vi "Main.vi"() -> ()   [LabVIEW 2019]
panel:
  out "status reference out":bool=TRUE
  in  "Find":bool
  in  "stop 2":bool
  in  "axis in":u8
  in  "stop":bool
  in  "Tab Control":enum32{"Navigation", "Interface", "About"}(tab)
  in  "find ref":bool
  in  "Reference Auto Update 3":bool=TRUE caption="Auto Update"
  out "move out":bool=TRUE caption="Move"
  in  "Positioner 2":u16(ring)=15 caption="Positioner" items=["ECGp5050", "ECGt5050", "ECR3030", "ECR4040", "ECR5050", "ECSx3030", "ECSx3040", "ECSx3050", "ECSx3060", "ECSx3070", "ECSx3080", "ECSx5050", "ECSxy5050", "ECSz3030", "ECSz5050", "EOP1", "EOP2", "EOP3"]
  out "in target range3":bool
  in  "auto Reset 1":bool=TRUE caption="Auto Reset"
  in  "Target Range 3":u32 caption="Target Range"
  in  "Reset Error 2":bool
  in  "Reset Error 3":bool
  out "Error 3":bool caption="Error"
  out "Error Message 3":string
  out "actor type 2":u16(ring) caption="Status" items=["linear positioner"=0, "rotator"=1, "goniometer"=2, "< error >"=9]
  out "actor type":u16(ring) caption="Status" items=["linear positioner"=0, "rotator"=1, "goniometer"=2, "< error >"=9]
  out "EotLeftDetected3":bool caption="Status Eot BWD"
  out "EotrightDetected3":bool caption="Status Eot FWD"
  in  "EoT 3":bool=TRUE caption="Stop on EoT"
  out "EotLeftDetected2":bool caption="Status Eot BWD"
  out "EotrightDetected2":bool caption="Status Eot FWD"
  in  "EoT 2":bool=TRUE caption="Stop on EoT"
  in  "Move 3":bool
  out "MoveSignal 3":bool caption="Positioner Connected/Moving"
  out "MoveSignal":bool caption="Positioner Connected/Moving"
  out "ReferenceSignal":bool=TRUE
  in  "Axis 3":bool caption="Closed Loop Funktions"
  in  "Axis 2":bool caption="Closed Loop Funktions"
  in  "Target Position 3":i32 caption="Target Position [µm]"
  in  "Target Position 1":i32 caption="Target position [µm]"
  in  "Number of steps 3":i32=1 caption="Number of Steps"
  in  "Number of steps 2":i32=1 caption="Number of Steps"
  in  "Output 2":bool caption="Axis 2"
  in  "Move 2":bool
  in  "Move":bool
  out "ReferenceSignal 3":bool
  out "Reference 3":dbl caption="Reference position [nm]" format="%#_6f"
  in  "Output":bool=TRUE caption="Axis 1"
  out "Output Satus 3":bool caption="Output Status"
  in  "Reference Auto Update 2":bool=TRUE caption="Auto Update"
  out "Error Message":string
  out "Error":bool
  in  "Output 3":bool caption="Axis 3"
  in  "auto Reset 3":bool=TRUE caption="Auto Reset"
  out "Output Status 1":bool=TRUE caption="Output Status"
  out "Position 3":dbl caption="Position [nm]" format="%#_6f"
  out "Output Status 2":bool caption="Output Status"
  in  "amplitude [V] 3":dbl=45.001 caption="Amplitude [V]" format="%#.3f"
  in  "frequency [Hz] 3":dbl=997.363 caption="Frequency [Hz]" format="%#.3f"
  out "Error 2":bool caption="Error"
  out "actor type 3":u16(ring) caption="Status" items=["linear positioner"=0, "rotator"=1, "goniometer"=2, "< error >"=9]
  out "Error Message 2":string
  out "Connected 3":bool caption="Connected"
  in  "Single Step Left 3":bool caption="Open Loop Funktions"
  in  "Positioner 3":u16(ring)=15 caption="Positioner" items=["ECGp5050", "ECGt5050", "ECR3030", "ECR4040", "ECR5050", "ECSx3030", "ECSx3040", "ECSx3050", "ECSx3060", "ECSx3070", "ECSx3080", "ECSx5050", "ECSxy5050", "ECSz3030", "ECSz5050", "EOP1", "EOP2", "EOP3"]
  in  "Endless Left 3":bool caption="Continuous Backward"
  in  "Continuous Forward":bool
  in  "Single Step Right 3":bool caption="Step(s)"
  in  "Fixed DC 3":i32 caption="DC Level [mV]"
  out "move out 3":bool=TRUE caption="Move"
  out "Position 2":dbl caption="Position [nm]" format="%#_6f"
  in  "amplitude [V] 2":dbl=45.001 caption="Amplitude [V]" format="%#.3f"
  in  "Amplitude [V]":dbl=45.001 format="%#.3f"
  in  "frequency [Hz] 2":dbl=997.363 caption="Frequency [Hz]" format="%#.3f"
  in  "Frequency [Hz]":dbl=1998.531 format="%#.3f"
  out "Connected 2":bool caption="Connected"
  in  "Single Step Left":bool caption="Open Loop Funktions"
  in  "Single Step Left 2":bool caption="Open Loop Funktions"
  in  "Single Step Right 2":bool caption="Step(s)"
  in  "Number of steps 1":i32=1 caption="Number of Steps"
  out "ReferenceSignal 2":bool
  in  "Single Step Right":bool caption="Step(s)"
  in  "Endless Left":bool caption="Continuous Backward"
  in  "Continuous Forward":bool
  in  "Endless Left 2":bool caption="Continuous Backward"
  out "EotLeftDetected1":bool caption="Status Eot BWD"
  out "EotrightDetected1":bool caption="Status Eot FWD"
  in  "EoT 1":bool caption="Stop on EoT"
  in  "Target position 2":i32 caption="Target Position [µm]"
  out "in target range2":bool
  in  "Continuous Forward":bool
  out "Reference 2":dbl caption="Reference position [nm]" format="%#_6f"
  in  "Fixed DC 2":i32 caption="DC Level [mV]"
  out "MoveSignal 2":bool caption="Positioner Connected/Moving"
  out "in target range1":bool
  in  "Target Range 2":u32 caption="Target Range [nm]"
  in  "Target Range 1":u32 caption="Target Range"
  out "Reference":dbl=-7597148.0 caption="Reference position [nm]" format="%#_6f"
  in  "auto Reset 2":bool=TRUE caption="Auto Reset"
  out "Position":dbl=14701.126 caption="Position [nm]" format="%#_6f"
  in  "Axis 1":bool caption="Closed Loop Funktions"
  in  "Fixed DC 1":i32 caption="DC Level [mV]"
  out "move out 2":bool=TRUE caption="Move"
  in  "Reset Error":bool
  out "Connected":bool=TRUE
  in  "Positioner":u16(ring)=15 items=["ECGp5050", "ECGt5050", "ECR3030", "ECR4040", "ECR5050", "ECSx3030", "ECSx3040", "ECSx3050", "ECSx3060", "ECSx3070", "ECSx3080", "ECSx5050", "ECSxy5050", "ECSz3030", "ECSz5050", "EOP1", "EOP2", "EOP3"]
  in  "Reference Auto Update 1":bool=TRUE caption="Auto Update"
  out "Voltage (mv)":i64
  out "Error 4":bool caption="Error"
  out "Error Message 4":string
  in  "Mode Input 1":u16(ring) caption="Mode" items=["Trigger (LVDS)"=11, "Trigger (LVTTL)"=10, "Stepper (LVDS)"=9, "Stepper (LVTTL)"=8, "AquadB (LVDS)"=1, "AquadB (LVTTL)"=0, "OFF"=15]
  in  "Loop Mode 1":u16(ring) caption="Loop mode" items=["closed-loop"=1, "open-loop"=0]
  in  "Steps per pulse 1":i32 caption="Steps per pulse [Steps]"
  in  "Change per pulse 1":i32 caption="Change per pulse [u°/nm]"
  out "RT in move Signal 1":bool=TRUE caption="move"
  in  "RT in move 1":bool=TRUE caption="Move"
  in  "AquadB in res 1":i32 caption="AquadB Resolution [nm]"
  in  "AquadB out 1":bool caption="AquadB enable"
  in  "AqaudB clock 1":i32 caption="AquadB Clock [ns]"
  in  "AquadB Resolution 1":i32 caption="AquadB Resolution [nm]"
  in  "Reset Error 4":bool
  out "Error 5":bool caption="Error"
  out "Error Message 5":string
  in  "Mode Input 2":u16(ring) caption="Mode" items=["Trigger (LVDS)"=11, "Trigger (LVTTL)"=10, "Stepper (LVDS)"=9, "Stepper (LVTTL)"=8, "AquadB (LVDS)"=1, "AquadB (LVTTL)"=0, "OFF"=15]
  in  "Loop Mode 2":u16(ring) caption="Loop mode" items=["closed-loop"=1, "open-loop"=0]
  in  "Steps per pulse 2":i32 caption="Steps per pulse [Steps]"
  in  "Change per pulse 2":i32 caption="Change per pulse  [u°/nm]"
  out "RT in move Signal 2":bool=TRUE caption="move"
  in  "RT in move 2":bool=TRUE caption="Move"
  in  "AquadB in res 2":i32 caption="AquadB Resolution [nm]"
  in  "AquadB out 2":bool caption="AquadB enable"
  in  "AqaudB clock 2":i32 caption="AquadB Clock [ns]"
  in  "AquadB Resolution 2":i32 caption="AquadB Resolution [nm]"
  in  "Reset Error 5":bool
  out "Error 6":bool caption="Error"
  out "Error Message 6":string
  in  "Mode Input 3":u16(ring) caption="Mode" items=["Trigger (LVDS)"=11, "Trigger (LVTTL)"=10, "Stepper (LVDS)"=9, "Stepper (LVTTL)"=8, "AquadB (LVDS)"=1, "AquadB (LVTTL)"=0, "OFF"=15]
  in  "Loop Mode 3":u16(ring) caption="Loop mode" items=["closed-loop"=1, "open-loop"=0]
  in  "Steps per pulse 3":i32 caption="Steps per pulse [Steps]"
  in  "Change per pulse 3":i32 caption="Change per pulse  [u°/nm]"
  out "RT in move Signal 3":bool=TRUE caption="move"
  in  "RT in move 3":bool=TRUE caption="Move"
  in  "AquadB in res 3":i32 caption="AquadB Resolution [nm]"
  in  "Output Mode":u16(ring) caption="Mode" items=["AquadB (LVTTL)", "AquadB (LVDS)"]
  in  "AquadB out 3":bool caption="AquadB enable"
  in  "AqaudB clock 3":i32 caption="AquadB Clock [ns]"
  in  "AquadB Resolution 3":i32 caption="AquadB Resolution [nm]"
  in  "Reset Error 6":bool
  in  "Reboot":bool
  in  "Factory Reset":bool
  in  "Reset Error 8":bool
  out "Error Message 7":string
  in  "Lock password":string
  in  "name":string="Test" caption="Device Name"
  in  "Access Password":string
  out "Error 7":bool caption="Error"
  out "locked":bool
  out "authorized":bool
  in  "Unlock":bool=TRUE
  out "Name":string caption="Device Name"
  out "Device type":string="AMC100/NUM"
  out "Sn":string caption="Serial Number"
  out "ip":string="192.168.1.1" caption="IP Adress"
  out "Firmware Version":string
  out "FPGA Version":string
  out "Mac Adress":string
  # "Real Time Input"
  # "Real Time Output"
  # "Global Parameters"
  # "Axis 1"
  # "Axis 1"
  # "Axis 2"
  # "Axis 2"
  # "Axis 3"
  # "Axis 3"
  # "Device Info"
  # "Device Access"
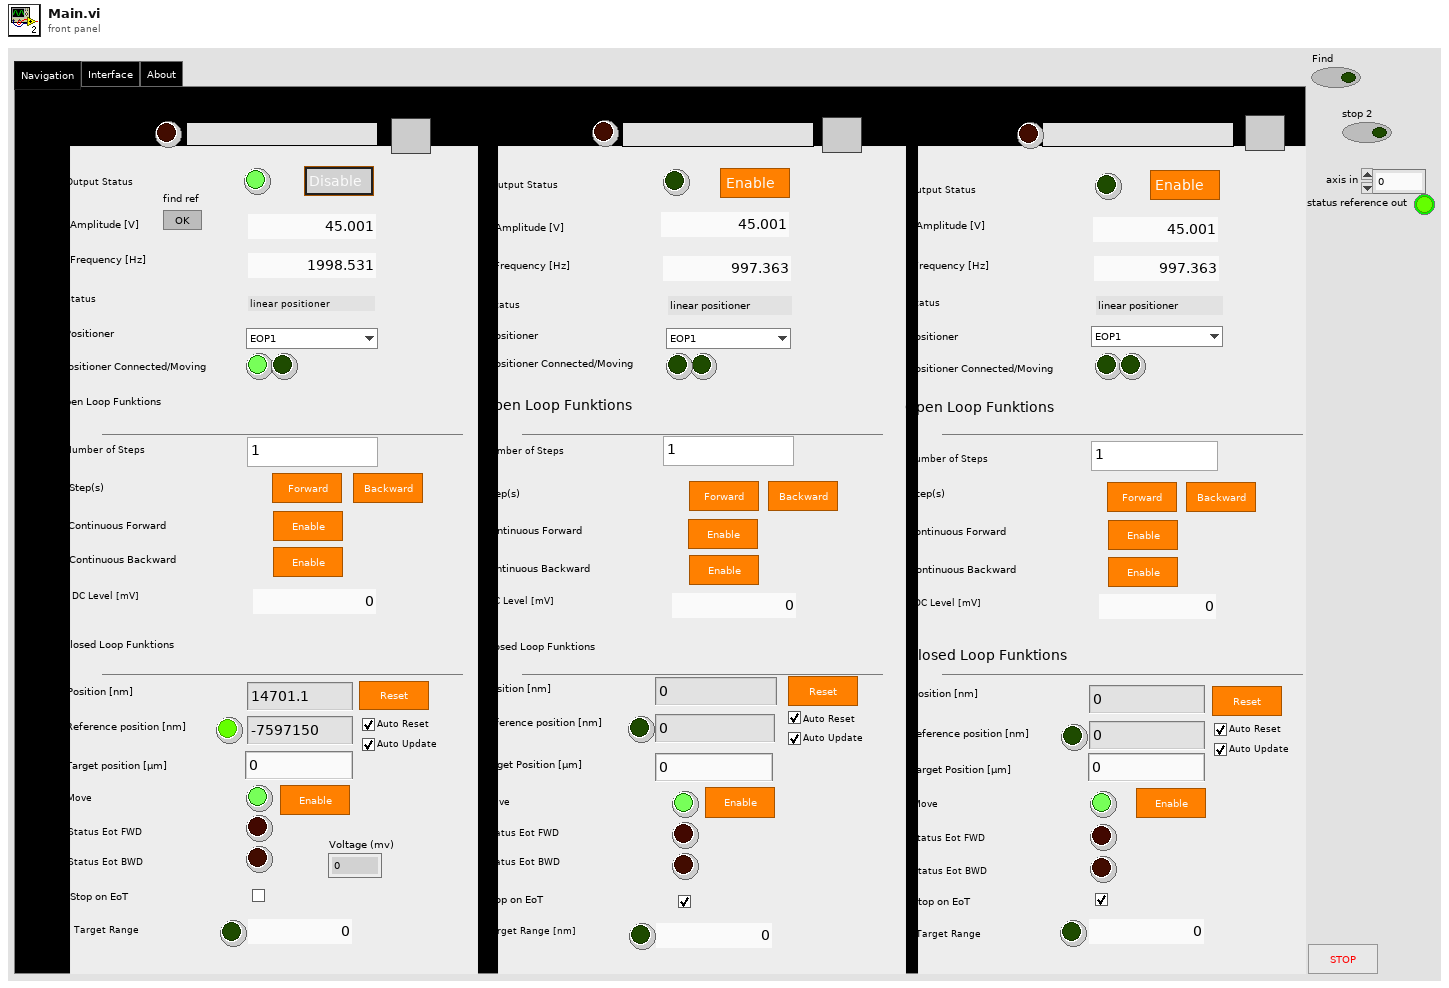
[diagram p1: front panel]
types:
  T1 = enum8{"Enabled", "Disabled", "Disabled and Grayed Out"}
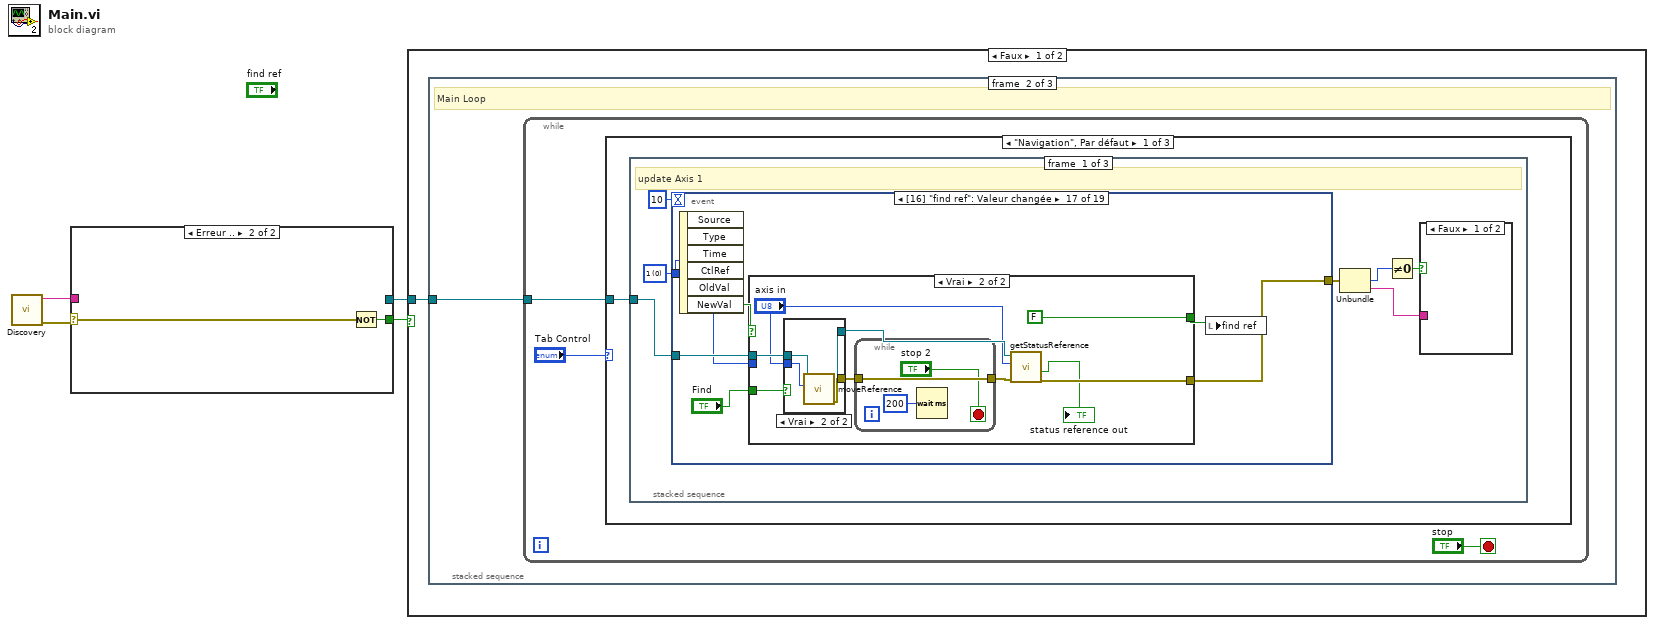
[diagram p0: block diagram]
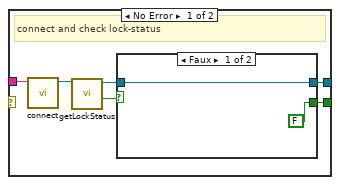
[diagram p2: hidden frame]
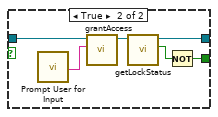
[diagram p3: hidden frame]
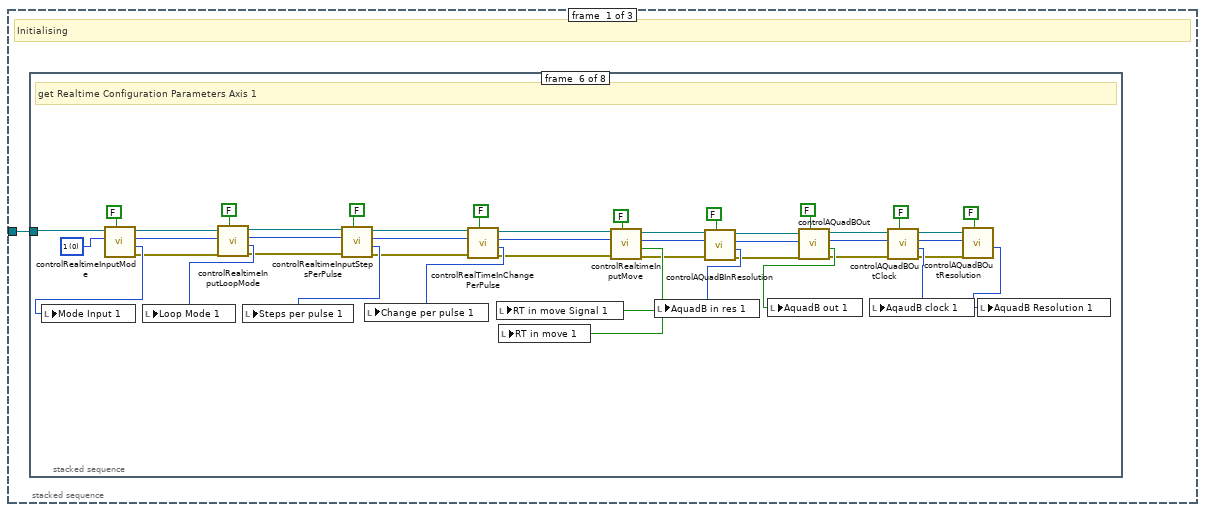
[diagram p4: hidden frame]
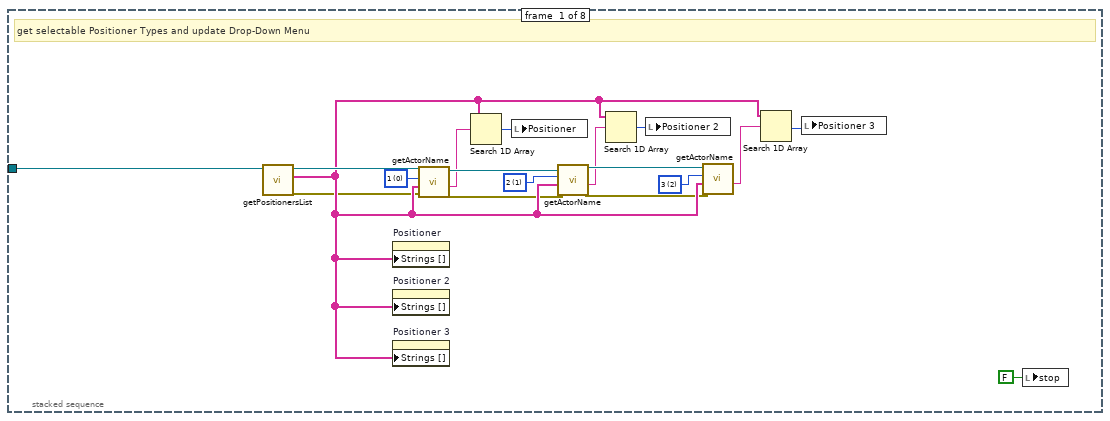
[diagram p5: hidden frame]
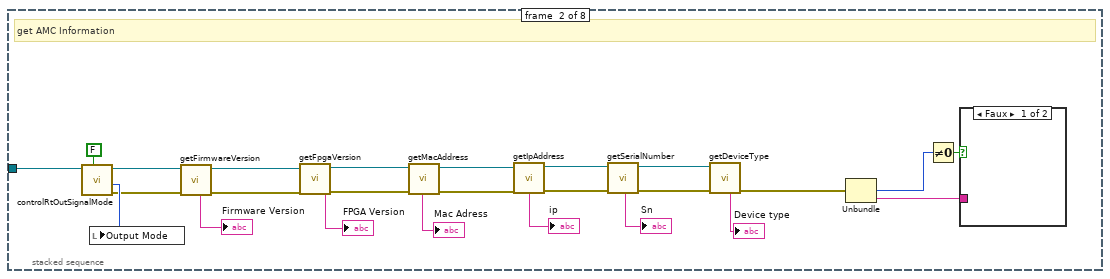
[diagram p6: hidden frame]
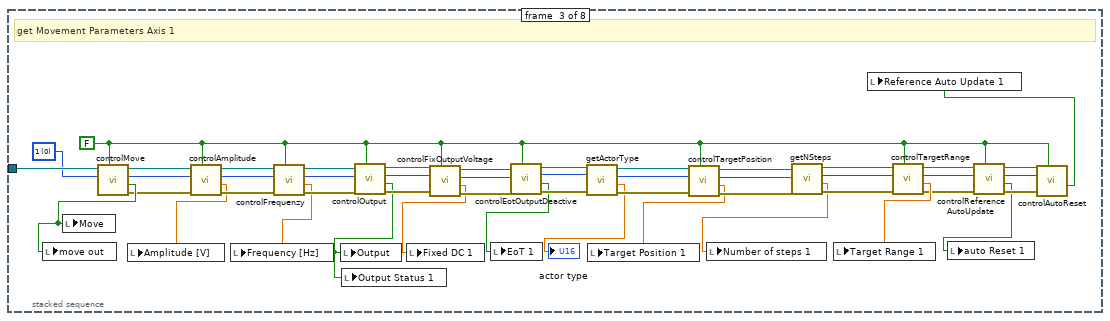
[diagram p8: hidden frame]
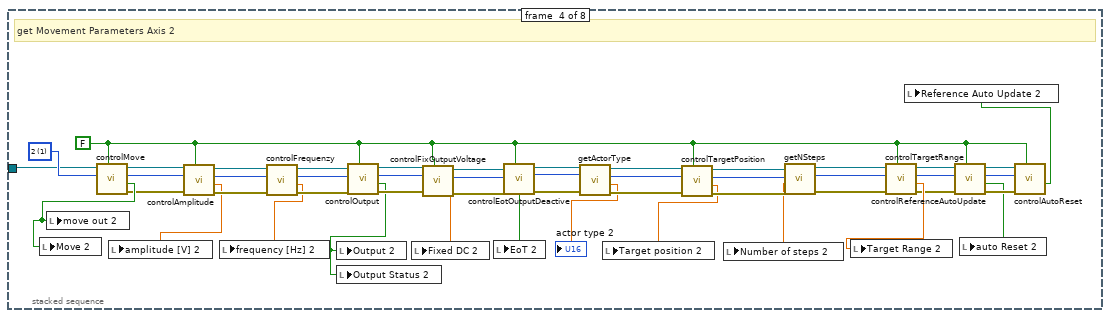
[diagram p9: hidden frame]
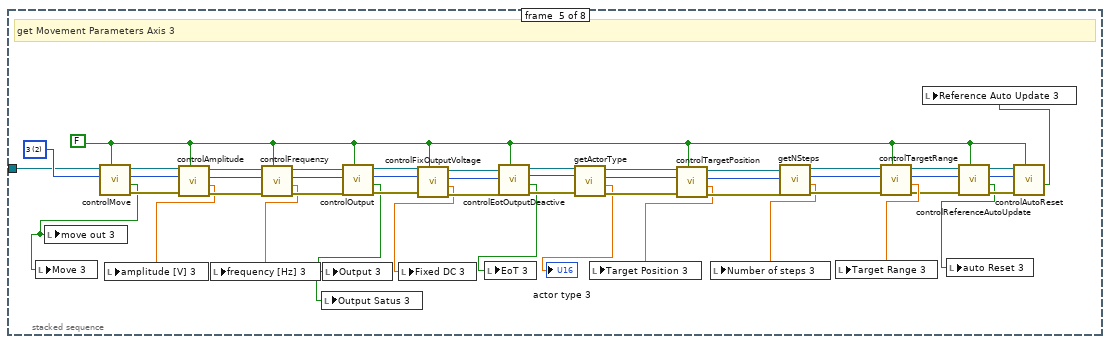
[diagram p10: hidden frame]
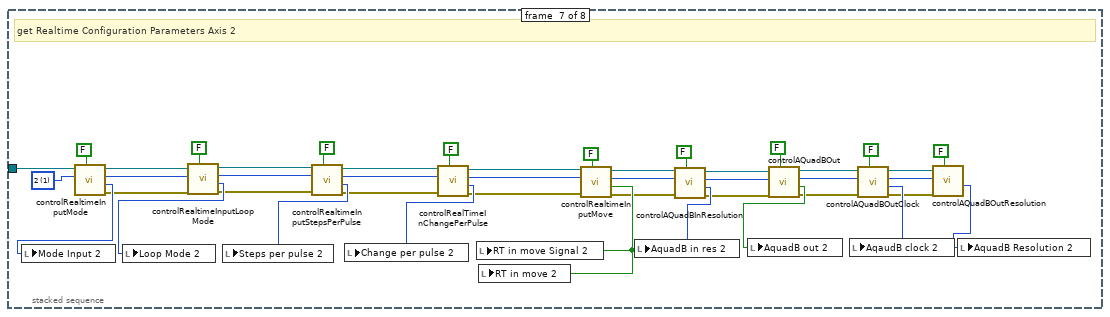
[diagram p11: hidden frame]
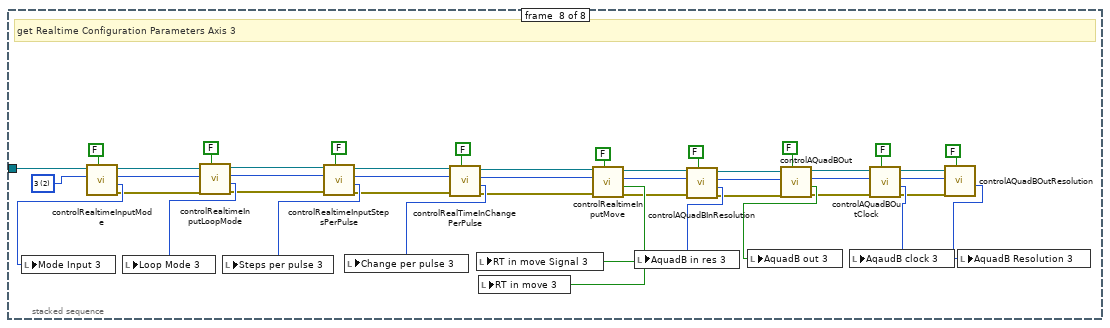
[diagram p12: hidden frame]
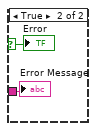
[diagram p13: hidden frame]
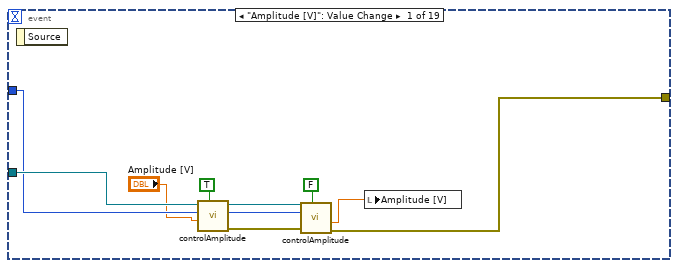
[diagram p14: hidden frame]
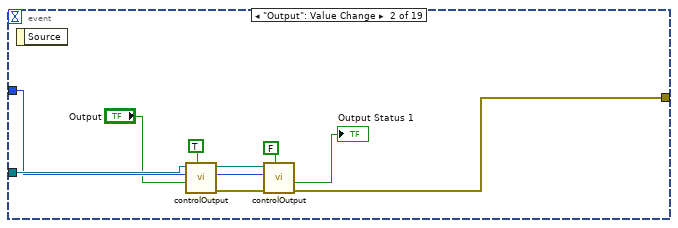
[diagram p15: hidden frame]
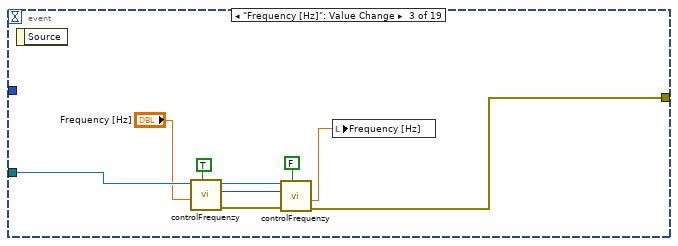
[diagram p16: hidden frame]
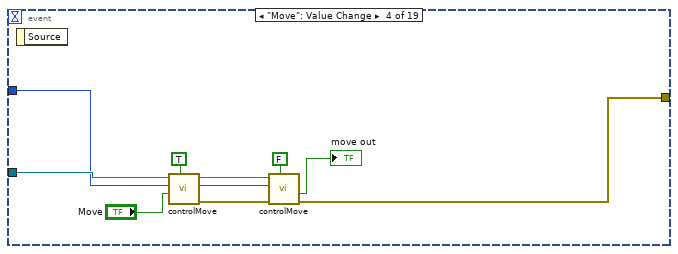
[diagram p17: hidden frame]
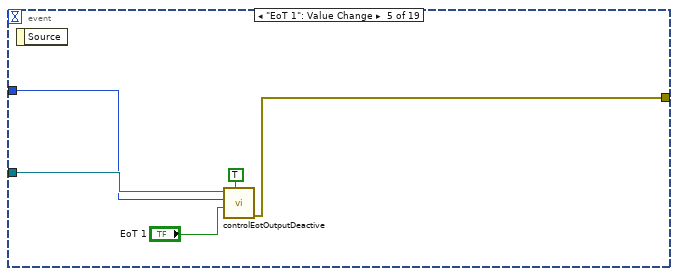
[diagram p18: hidden frame]
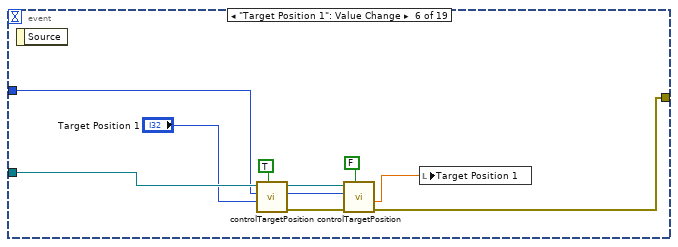
[diagram p19: hidden frame]
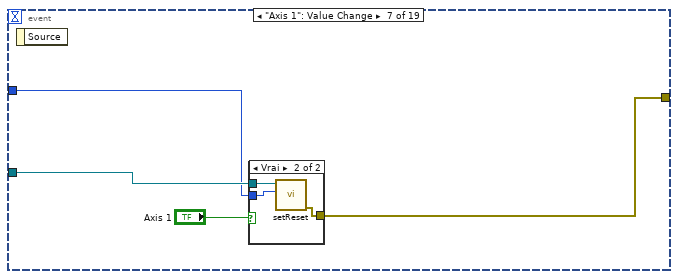
[diagram p20: hidden frame]
diagram:
  n1 = call "Discovery.vi"() -> ("error out"=w2:errorcluster, "IP"=w1:string)  [unwired: 10 in]
  n2 = case shown="Erreur .." w2 {
    selector: w2 -> [_ w19]
    tunnel: [w10 w20] -> w4
    tunnel: [w9 _] -> w3
    tunnel: w1 -> [w5 _]
    frame No Error {
      # "connect and check lock-status"
      n3 = call "connect.vi"("deviceAddress"=w5) -> ("connection ID"=w8:refnum<k5>)  [unwired: 5 in, 1 out]
      n4 = call "getLockStatus.vi"("connection ID in"=w8) -> ("locked"=w6:bool, "connection ID out"=w7:refnum<k5>)  [unwired: 7 in, 2 out]
      n5 = case shown="Faux" w6 {
        tunnel: w7 -> [w12 w18]
        tunnel: [w12 w15] -> w9
        tunnel: [FALSE w14] -> w10
        frame False {
        }
        frame True {
          n6 = call "Prompt User for Input"() -> ("password"=w17:string)  [unwired: 17 in, 2 out]
          n7 = call "grantAccess.vi"("password"=w17, "connection ID"=w18) -> ("connection ID"=w16:refnum<k5>)  [unwired: 8 in, 1 out]
          n8 = call "getLockStatus.vi"("connection ID in"=w16) -> ("authorized"=w13:bool, "connection ID out"=w15:refnum<k5>)  [unwired: 7 in, 2 out]
          n9 = Not(x=w13) -> (.not. x?=w14:bool)
        }
      }
    }
    frame Error {
      n10 = Not(x=w19) -> (.not. x?=w20:bool)
    }
  }
  n11 = case shown="Faux" w4 {
    tunnel: w3 -> [w21 _]
    frame False {
      n12 = stacked-sequence {
        tunnel: w21 -> [w22 w342 w1357]
        frame #0 {
          # "Initialising"
          n13 = stacked-sequence {
            tunnel: w22 -> [w40 w44 w72 w120 w166 w253 w297 w341]
            frame #0 {
              w37 = u8 2 items=["1", "2", "3"] ("axis")
              w34 = u8 1 items=["1", "2", "3"] ("axis")
              w31 = u8 0 items=["1", "2", "3"] ("axis")
              # "get selectable Positioner Types and update Drop-Down Menu"
              n14 = call "getPositionersList.vi"("connection ID"=w40) -> ("error out"=w23:errorcluster, "Positioners List"=w26:string[], "connection ID"=w30:refnum<k5>)  [unwired: 8 in]
              n15 = property on="Positioner" class="MDér (strict)"("Strings []"=w26) -> ()  [unwired: 2 in, 2 out]
              n16 = property on="Positioner 2" class="MDér (strict)"("Strings []"=w26) -> ()  [unwired: 2 in, 2 out]
              n17 = property on="Positioner 3" class="MDér (strict)"("Strings []"=w26) -> ()  [unwired: 2 in, 2 out]
              n18 = call "getActorName.vi"("error in"=w23, "Actor Names"=w26, "axis in"=w31, "connection ID"=w30) -> ("error out"=w25:errorcluster, "ActorName out"=w32:string, "connection ID"=w33:refnum<k5>)  [unwired: 4 in, 1 out]
              n19 = Search 1D Array(1D array=w26, element=w32) -> (index of element=w27:i32)  [unwired: 1 in]
              n20 = local write "Positioner"(w27) -> ()
              n21 = call "getActorName.vi"("error in"=w25, "Actor Names"=w26, "axis in"=w34, "connection ID"=w33) -> ("error out"=w24:errorcluster, "ActorName out"=w35:string, "connection ID"=w36:refnum<k5>)  [unwired: 4 in, 1 out]
              n22 = Search 1D Array(1D array=w26, element=w35) -> (index of element=w28:i32)  [unwired: 1 in]
              n23 = local write "Positioner 2"(w28) -> ()
              n24 = call "getActorName.vi"("error in"=w24, "Actor Names"=w26, "axis in"=w37, "connection ID"=w36) -> ("ActorName out"=w38:string)  [unwired: 4 in, 3 out]
              n25 = Search 1D Array(1D array=w26, element=w38) -> (index of element=w29:i32)  [unwired: 1 in]
              n26 = local write "Positioner 3"(w29) -> ()
              n27 = local write "stop"(FALSE ("stop")) -> ()
            }
            frame #1 {
              # "get AMC Information"
              n28 = call "controlRtOutSignalMode.vi"("Set"=FALSE, "connection ID"=w44) -> ("error out"=w42:errorcluster, "RT out Mode out"=w45:i32, "connection ID"=w43:refnum<k5>)  [unwired: 7 in]
              n29 = local write "Output Mode"(w45) -> ()
              n30 = call "getFirmwareVersion.vi"("error in"=w42, "connection ID"=w43) -> ("error out"=w51:errorcluster, "Firmware Version out"=→"Firmware Version":string, "connection ID"=w61:refnum<k5>)  [unwired: 7 in]
              n31 = call "getFpgaVersion.vi"("error in"=w51, "connection ID"=w61) -> ("error out"=w50:errorcluster, "FPGA out"=→"FPGA Version":string, "connection ID"=w59:refnum<k5>)  [unwired: 7 in]
              n32 = call "getMacAddress.vi"("error in"=w50, "connection ID"=w59) -> ("error out"=w49:errorcluster, "Mac Adress out"=→"Mac Adress":string, "connection ID"=w56:refnum<k5>)  [unwired: 7 in]
              n33 = call "getIpAddress.vi"("error in"=w49, "connection ID"=w56) -> ("error out"=w48:errorcluster, "IP out"=→"ip":string, "connection ID"=w55:refnum<k5>)  [unwired: 7 in]
              n34 = call "getSerialNumber.vi"("error in"=w48, "connection ID"=w55) -> ("error out"=w47:errorcluster, "sn out"=→"Sn":string, "connection ID"=w53:refnum<k5>)  [unwired: 7 in]
              n35 = call "getDeviceType.vi"("error in"=w47, "connection ID"=w53) -> ("error out"=w41:errorcluster, "Device Type out"=→"Device type":string)  [unwired: 7 in, 1 out]
              n36 = Unbundle(w41) -> ("code"=w64:i32, "source"=w65:string)  [unwired: 1 out]
              n37 = Not Equal To 0?(x=w64) -> (x != 0?=w63:bool)
              n38 = case shown="Faux" w63 {
                tunnel: w65 -> [_ _]
                frame False {
                }
                frame True {
                }
              }
            }
            frame #2 {
              w70 = u8 0 items=["1", "2", "3"] ("axis")
              w73 = FALSE ("set")
              # "get Movement Parameters Axis 1"
              n39 = call "controlMove.vi"("Set"=w73, "axis in"=w70, "connection ID"=w72) -> ("error out"=w67:errorcluster, "controll move out"=w68:bool, "axis out"=w69:u8, "connection ID"=w71:refnum<k5>)  [unwired: 5 in]
              n40 = local write "move out"(w68) -> ()
              n41 = local write "Move"(w68) -> ()
              n42 = call "controlAmplitude.vi"("Set"=w73, "error in"=w67, "axis in"=w69, "connection ID"=w71) -> ("error out"=w111:errorcluster, "amplitude [V] out"=w89:dbl, "axis out"=w113:u8, "connection ID"=w112:refnum<k5>)  [unwired: 4 in]
              n43 = local write "Amplitude [V]"(w89) -> ()
              n44 = call "controlFrequenzy.vi"("Set"=w73, "error in"=w111, "axis in"=w113, "connection ID"=w112) -> ("error out"=w108:errorcluster, "Frequenzy [Hz] out"=w88:dbl, "axis out"=w109:u8, "connection ID"=w110:refnum<k5>)  [unwired: 4 in]
              n45 = local write "Frequency [Hz]"(w88) -> ()
              n46 = call "controlOutput.vi"("Set"=w73, "error in"=w108, "axis in"=w109, "connection ID"=w110) -> ("error out"=w105:errorcluster, "enable output out"=w66:bool, "axis out"=w106:u8, "connection ID"=w107:refnum<k5>)  [unwired: 4 in]
              n47 = local write "Output"(w66) -> ()
              n48 = local write "Output Status 1"(w66) -> ()
              n49 = call "controlFixOutputVoltage.vi"("Set"=w73, "error in"=w105, "axis in"=w106, "connection ID"=w107) -> ("error out"=w102:errorcluster, "Fixed Output Voltage out"=w87:dbl, "axis out"=w103:u8, "connection ID"=w104:refnum<k5>)  [unwired: 4 in]
              n50 = local write "Fixed DC 1"(w87) -> ()
              n51 = call "controlEotOutputDeactive.vi"("Set"=w73, "error in"=w102, "axis in"=w103, "connection ID"=w104) -> ("error out"=w99:errorcluster, "enable EOT out"=w86:bool, "axis out"=w100:u8, "connection ID"=w101:refnum<k5>)  [unwired: 4 in]
              n52 = local write "EoT 1"(w86) -> ()
              n53 = call "getActorType.vi"("error in"=w99, "axis in"=w100, "connection ID"=w101) -> ("error out"=w96:errorcluster, "Actor Type"=→"actor type":dbl, "axis out"=w97:u8, "connection ID"=w98:refnum<k5>)  [unwired: 5 in]
              n54 = call "controlTargetPosition.vi"("Set"=w73, "error in"=w96, "axis in"=w97, "connection ID"=w98) -> ("error out"=w93:errorcluster, "Target Position out"=w84:dbl, "axis out"=w94:u8, "connection ID"=w95:refnum<k5>)  [unwired: 4 in]
              n55 = local write "Target Position 1"(w84) -> ()
              n56 = call "getNSteps.vi"("error in"=w93, "axis in"=w94, "connection ID"=w95) -> ("error out"=w90:errorcluster, "setnSteps out"=w83:dbl, "axis out"=w91:u8, "connection ID"=w92:refnum<k5>)  [unwired: 5 in]
              n57 = local write "Number of steps 1"(w83) -> ()
              n58 = call "controlTargetRange.vi"("Set"=w73, "error in"=w90, "axis in"=w91, "connection ID"=w92) -> ("error out"=w79:errorcluster, "Target Range out"=w82:dbl, "axis out"=w80:u8, "connection ID"=w81:refnum<k5>)  [unwired: 4 in]
              n59 = local write "Target Range 1"(w82) -> ()
              n60 = call "controlReferenceAutoUpdate.vi"("Set"=w73, "error in"=w79, "axis in"=w80, "connection ID"=w81) -> ("error out"=w76:errorcluster, "ref auto up out"=w75:bool, "axis out"=w77:u8, "connection ID"=w78:refnum<k5>)  [unwired: 4 in]
              n61 = local write "auto Reset 1"(w75) -> ()
              n62 = call "controlAutoReset.vi"("Set"=w73, "error in"=w76, "axis in"=w77, "connection ID"=w78) -> ("auto reset out"=w74:bool)  [unwired: 4 in, 3 out]
              n63 = local write "Reference Auto Update 1"(w74) -> ()
            }
            frame #3 {
              w121 = u8 1 items=["1", "2", "3"] ("axis")
              w114 = FALSE ("set")
              # "get Movement Parameters Axis 2"
              n64 = call "controlMove.vi"("Set"=w114, "axis in"=w121, "connection ID"=w120) -> ("error out"=w116:errorcluster, "controll move out"=w119:bool, "axis out"=w117:u8, "connection ID"=w118:refnum<k5>)  [unwired: 5 in]
              n65 = local write "Move 2"(w119) -> ()
              n66 = local write "move out 2"(w119) -> ()
              n67 = call "controlAmplitude.vi"("Set"=w114, "error in"=w116, "axis in"=w117, "connection ID"=w118) -> ("error out"=w159:errorcluster, "amplitude [V] out"=w137:dbl, "axis out"=w161:u8, "connection ID"=w160:refnum<k5>)  [unwired: 4 in]
              n68 = local write "amplitude [V] 2"(w137) -> ()
              n69 = call "controlFrequenzy.vi"("error in"=w159, "axis in"=w161, "connection ID"=w160) -> ("error out"=w156:errorcluster, "Frequenzy [Hz] out"=w136:dbl, "axis out"=w157:u8, "connection ID"=w158:refnum<k5>)  [unwired: 5 in]
              n70 = local write "frequency [Hz] 2"(w136) -> ()
              n71 = call "controlOutput.vi"("Set"=w114, "error in"=w156, "axis in"=w157, "connection ID"=w158) -> ("error out"=w153:errorcluster, "enable output out"=w115:bool, "axis out"=w154:u8, "connection ID"=w155:refnum<k5>)  [unwired: 4 in]
              n72 = local write "Output 2"(w115) -> ()
              n73 = local write "Output Status 2"(w115) -> ()
              n74 = call "controlFixOutputVoltage.vi"("Set"=w114, "error in"=w153, "axis in"=w154, "connection ID"=w155) -> ("error out"=w150:errorcluster, "Fixed Output Voltage out"=w135:dbl, "axis out"=w151:u8, "connection ID"=w152:refnum<k5>)  [unwired: 4 in]
              n75 = local write "Fixed DC 2"(w135) -> ()
              n76 = call "controlEotOutputDeactive.vi"("Set"=w114, "error in"=w150, "axis in"=w151, "connection ID"=w152) -> ("error out"=w147:errorcluster, "enable EOT out"=w134:bool, "axis out"=w148:u8, "connection ID"=w149:refnum<k5>)  [unwired: 4 in]
              n77 = local write "EoT 2"(w134) -> ()
              n78 = call "getActorType.vi"("error in"=w147, "axis in"=w148, "connection ID"=w149) -> ("error out"=w144:errorcluster, "Actor Type"=→"actor type 2":dbl, "axis out"=w145:u8, "connection ID"=w146:refnum<k5>)  [unwired: 5 in]
              n79 = call "controlTargetPosition.vi"("Set"=w114, "error in"=w144, "axis in"=w145, "connection ID"=w146) -> ("error out"=w141:errorcluster, "Target Position out"=w132:dbl, "axis out"=w142:u8, "connection ID"=w143:refnum<k5>)  [unwired: 4 in]
              n80 = local write "Target position 2"(w132) -> ()
              n81 = call "getNSteps.vi"("error in"=w141, "axis in"=w142, "connection ID"=w143) -> ("error out"=w138:errorcluster, "setnSteps out"=w131:dbl, "axis out"=w139:u8, "connection ID"=w140:refnum<k5>)  [unwired: 5 in]
              n82 = local write "Number of steps 2"(w131) -> ()
              n83 = call "controlTargetRange.vi"("Set"=w114, "error in"=w138, "axis in"=w139, "connection ID"=w140) -> ("error out"=w125:errorcluster, "Target Range out"=w130:dbl, "axis out"=w127:u8, "connection ID"=w129:refnum<k5>)  [unwired: 4 in]
              n84 = local write "Target Range 2"(w130) -> ()
              n85 = call "controlReferenceAutoUpdate.vi"("Set"=w114, "error in"=w125, "axis in"=w127, "connection ID"=w129) -> ("error out"=w124:errorcluster, "ref auto up out"=w123:bool, "axis out"=w126:u8, "connection ID"=w128:refnum<k5>)  [unwired: 4 in]
              n86 = local write "auto Reset 2"(w123) -> ()
              n87 = call "controlAutoReset.vi"("Set"=w114, "error in"=w124, "axis in"=w126, "connection ID"=w128) -> ("auto reset out"=w122:bool)  [unwired: 4 in, 3 out]
              n88 = local write "Reference Auto Update 2"(w122) -> ()
            }
            frame #4 {
              w167 = u8 2 items=["1", "2", "3"] ("axis")
              w165 = FALSE ("set")
              # "get Movement Parameters Axis 3"
              n89 = call "controlMove.vi"("Set"=w165, "axis in"=w167, "connection ID"=w166) -> ("error out"=w164:errorcluster, "controll move out"=w163:bool, "axis out"=w168:u8, "connection ID"=w169:refnum<k5>)  [unwired: 5 in]
              n90 = local write "Move 3"(w163) -> ()
              n91 = local write "move out 3"(w163) -> ()
              n92 = call "controlAmplitude.vi"("Set"=w165, "error in"=w164, "axis in"=w168, "connection ID"=w169) -> ("error out"=w207:errorcluster, "amplitude [V] out"=w185:dbl, "axis out"=w209:u8, "connection ID"=w208:refnum<k5>)  [unwired: 4 in]
              n93 = local write "amplitude [V] 3"(w185) -> ()
              n94 = call "controlFrequenzy.vi"("Set"=w165, "error in"=w207, "axis in"=w209, "connection ID"=w208) -> ("error out"=w204:errorcluster, "Frequenzy [Hz] out"=w184:dbl, "axis out"=w205:u8, "connection ID"=w206:refnum<k5>)  [unwired: 4 in]
              n95 = local write "frequency [Hz] 3"(w184) -> ()
              n96 = call "controlOutput.vi"("Set"=w165, "error in"=w204, "axis in"=w205, "connection ID"=w206) -> ("error out"=w201:errorcluster, "enable output out"=w162:bool, "axis out"=w202:u8, "connection ID"=w203:refnum<k5>)  [unwired: 4 in]
              n97 = local write "Output Satus 3"(w162) -> ()
              n98 = local write "Output 3"(w162) -> ()
              n99 = call "controlFixOutputVoltage.vi"("Set"=w165, "error in"=w201, "axis in"=w202, "connection ID"=w203) -> ("error out"=w198:errorcluster, "Fixed Output Voltage out"=w183:dbl, "axis out"=w199:u8, "connection ID"=w200:refnum<k5>)  [unwired: 4 in]
              n100 = local write "Fixed DC 3"(w183) -> ()
              n101 = call "controlEotOutputDeactive.vi"("Set"=w165, "error in"=w198, "axis in"=w199, "connection ID"=w200) -> ("error out"=w195:errorcluster, "enable EOT out"=w182:bool, "axis out"=w196:u8, "connection ID"=w197:refnum<k5>)  [unwired: 4 in]
              n102 = local write "EoT 3"(w182) -> ()
              n103 = call "getActorType.vi"("error in"=w195, "axis in"=w196, "connection ID"=w197) -> ("error out"=w192:errorcluster, "Actor Type"=→"actor type 3":dbl, "axis out"=w193:u8, "connection ID"=w194:refnum<k5>)  [unwired: 5 in]
              n104 = call "controlTargetPosition.vi"("Set"=w165, "error in"=w192, "axis in"=w193, "connection ID"=w194) -> ("error out"=w189:errorcluster, "Target Position out"=w181:dbl, "axis out"=w190:u8, "connection ID"=w191:refnum<k5>)  [unwired: 4 in]
              n105 = local write "Target Position 3"(w181) -> ()
              n106 = call "getNSteps.vi"("error in"=w189, "axis in"=w190, "connection ID"=w191) -> ("error out"=w186:errorcluster, "setnSteps out"=w180:dbl, "axis out"=w187:u8, "connection ID"=w188:refnum<k5>)  [unwired: 5 in]
              n107 = local write "Number of steps 3"(w180) -> ()
              n108 = call "controlTargetRange.vi"("Set"=w165, "error in"=w186, "axis in"=w187, "connection ID"=w188) -> ("error out"=w172:errorcluster, "Target Range out"=w179:dbl, "axis out"=w173:u8, "connection ID"=w174:refnum<k5>)  [unwired: 4 in]
              n109 = local write "Target Range 3"(w179) -> ()
              n110 = call "controlReferenceAutoUpdate.vi"("Set"=w165, "error in"=w172, "axis in"=w173, "connection ID"=w174) -> ("error out"=w175:errorcluster, "ref auto up out"=w171:bool, "axis out"=w176:u8, "connection ID"=w177:refnum<k5>)  [unwired: 4 in]
              n111 = local write "auto Reset 3"(w171) -> ()
              n112 = call "controlAutoReset.vi"("Set"=w165, "error in"=w175, "axis in"=w176, "connection ID"=w177) -> ("auto reset out"=w170:bool)  [unwired: 4 in, 3 out]
              n113 = local write "Reference Auto Update 3"(w170) -> ()
            }
            frame #5 {
              w211 = u8 0 items=["1", "2", "3"] ("axis")
              # "get Realtime Configuration Parameters Axis 1"
              n114 = call "controlRealtimeInputMode.vi"("Set"=FALSE, "axis in"=w211, "connection ID"=w253) -> ("error out"=w228:errorcluster, "RT Mode out"=w252:i32, "axis out"=w220:u8, "connection ID"=w212:refnum<k5>)  [unwired: 5 in]
              n115 = local write "Mode Input 1"(w252) -> ()
              n116 = call "controlRealtimeInputLoopMode.vi"("Set"=FALSE, "error in"=w228, "axis in"=w220, "connection ID"=w212) -> ("error out"=w229:errorcluster, "RT Loop out"=w251:i32, "axis out"=w221:u8, "connection ID"=w213:refnum<k5>)  [unwired: 4 in]
              n117 = local write "Loop Mode 1"(w251) -> ()
              n118 = call "controlRealtimeInputStepsPerPulse.vi"("Set"=FALSE, "error in"=w229, "axis in"=w221, "connection ID"=w213) -> ("error out"=w230:errorcluster, "Steps out"=w250:i32, "axis out"=w222:u8, "connection ID"=w214:refnum<k5>)  [unwired: 4 in]
              n119 = local write "Steps per pulse 1"(w250) -> ()
              n120 = call "controlRealTimeInChangePerPulse.vi"("Set"=FALSE, "error in"=w230, "axis in"=w222, "connection ID"=w214) -> ("error out"=w231:errorcluster, "Change out"=w249:i32, "axis out"=w223:u8, "connection ID"=w215:refnum<k5>)  [unwired: 4 in]
              n121 = local write "Change per pulse 1"(w249) -> ()
              n122 = call "controlRealtimeInputMove.vi"("Set"=FALSE, "error in"=w231, "axis in"=w223, "connection ID"=w215) -> ("error out"=w232:errorcluster, "move out"=w248:bool, "axis out"=w224:u8, "connection ID"=w216:refnum<k5>)  [unwired: 4 in]
              n123 = local write "RT in move Signal 1"(w248) -> ()
              n124 = local write "RT in move 1"(w248) -> ()
              n125 = call "controlAQuadBInResolution.vi"("Set"=FALSE, "error in"=w232, "axis in"=w224, "connection ID"=w216) -> ("error out"=w233:errorcluster, "Resolution out"=w247:i32, "axis out"=w225:u8, "connection ID"=w217:refnum<k5>)  [unwired: 3 in]
              n126 = local write "AquadB in res 1"(w247) -> ()
              n127 = call "controlAQuadBOut.vi"("Set"=FALSE, "error in"=w233, "axis in"=w225, "connection ID"=w217) -> ("error out"=w234:errorcluster, "ABout out"=w246:bool, "axis out"=w226:u8, "connection ID"=w218:refnum<k5>)  [unwired: 4 in]
              n128 = local write "AquadB out 1"(w246) -> ()
              n129 = call "controlAQuadBOutClock.vi"("Set"=FALSE, "error in"=w234, "axis in"=w226, "connection ID"=w218) -> ("error out"=w235:errorcluster, "clock out"=w245:i32, "axis out"=w227:u8, "connection ID"=w219:refnum<k5>)  [unwired: 4 in]
              n130 = local write "AqaudB clock 1"(w245) -> ()
              n131 = call "controlAQuadBOutResolution.vi"("Set"=FALSE, "error in"=w235, "axis in"=w227, "connection ID"=w219) -> ("ABoutRes out"=w244:i32)  [unwired: 4 in, 3 out]
              n132 = local write "AquadB Resolution 1"(w244) -> ()
            }
            frame #6 {
              w255 = u8 1 items=["1", "2", "3"] ("axis")
              # "get Realtime Configuration Parameters Axis 2"
              n133 = call "controlRealtimeInputMode.vi"("Set"=FALSE, "axis in"=w255, "connection ID"=w297) -> ("error out"=w272:errorcluster, "RT Mode out"=w296:i32, "axis out"=w264:u8, "connection ID"=w256:refnum<k5>)  [unwired: 5 in]
              n134 = local write "Mode Input 2"(w296) -> ()
              n135 = call "controlRealtimeInputLoopMode.vi"("Set"=FALSE, "error in"=w272, "axis in"=w264, "connection ID"=w256) -> ("error out"=w273:errorcluster, "RT Loop out"=w295:i32, "axis out"=w265:u8, "connection ID"=w257:refnum<k5>)  [unwired: 4 in]
              n136 = local write "Loop Mode 2"(w295) -> ()
              n137 = call "controlRealtimeInputStepsPerPulse.vi"("Set"=FALSE, "error in"=w273, "axis in"=w265, "connection ID"=w257) -> ("error out"=w274:errorcluster, "Steps out"=w294:i32, "axis out"=w266:u8, "connection ID"=w258:refnum<k5>)  [unwired: 4 in]
              n138 = local write "Steps per pulse 2"(w294) -> ()
              n139 = call "controlRealTimeInChangePerPulse.vi"("Set"=FALSE, "error in"=w274, "axis in"=w266, "connection ID"=w258) -> ("error out"=w275:errorcluster, "Change out"=w293:i32, "axis out"=w267:u8, "connection ID"=w259:refnum<k5>)  [unwired: 4 in]
              n140 = local write "Change per pulse 2"(w293) -> ()
              n141 = call "controlRealtimeInputMove.vi"("Set"=FALSE, "error in"=w275, "axis in"=w267, "connection ID"=w259) -> ("error out"=w276:errorcluster, "move out"=w292:bool, "axis out"=w268:u8, "connection ID"=w260:refnum<k5>)  [unwired: 4 in]
              n142 = local write "RT in move Signal 2"(w292) -> ()
              n143 = local write "RT in move 2"(w292) -> ()
              n144 = call "controlAQuadBInResolution.vi"("Set"=FALSE, "error in"=w276, "axis in"=w268, "connection ID"=w260) -> ("error out"=w277:errorcluster, "Resolution out"=w291:i32, "axis out"=w269:u8, "connection ID"=w261:refnum<k5>)  [unwired: 3 in]
              n145 = local write "AquadB in res 2"(w291) -> ()
              n146 = call "controlAQuadBOut.vi"("Set"=FALSE, "error in"=w277, "axis in"=w269, "connection ID"=w261) -> ("error out"=w278:errorcluster, "ABout out"=w290:bool, "axis out"=w270:u8, "connection ID"=w262:refnum<k5>)  [unwired: 4 in]
              n147 = local write "AquadB out 2"(w290) -> ()
              n148 = call "controlAQuadBOutClock.vi"("Set"=FALSE, "error in"=w278, "axis in"=w270, "connection ID"=w262) -> ("error out"=w279:errorcluster, "clock out"=w289:i32, "axis out"=w271:u8, "connection ID"=w263:refnum<k5>)  [unwired: 4 in]
              n149 = local write "AqaudB clock 2"(w289) -> ()
              n150 = call "controlAQuadBOutResolution.vi"("Set"=FALSE, "error in"=w279, "axis in"=w271, "connection ID"=w263) -> ("ABoutRes out"=w288:i32)  [unwired: 4 in, 3 out]
              n151 = local write "AquadB Resolution 2"(w288) -> ()
            }
            frame #7 {
              w299 = u8 2 items=["1", "2", "3"] ("axis")
              # "get Realtime Configuration Parameters Axis 3"
              n152 = call "controlRealtimeInputMode.vi"("Set"=FALSE, "axis in"=w299, "connection ID"=w341) -> ("error out"=w316:errorcluster, "RT Mode out"=w340:i32, "axis out"=w308:u8, "connection ID"=w300:refnum<k5>)  [unwired: 5 in]
              n153 = local write "Mode Input 3"(w340) -> ()
              n154 = call "controlRealtimeInputLoopMode.vi"("Set"=FALSE, "error in"=w316, "axis in"=w308, "connection ID"=w300) -> ("error out"=w317:errorcluster, "RT Loop out"=w339:i32, "axis out"=w309:u8, "connection ID"=w301:refnum<k5>)  [unwired: 4 in]
              n155 = local write "Loop Mode 3"(w339) -> ()
              n156 = call "controlRealtimeInputStepsPerPulse.vi"("Set"=FALSE, "error in"=w317, "axis in"=w309, "connection ID"=w301) -> ("error out"=w318:errorcluster, "Steps out"=w338:i32, "axis out"=w310:u8, "connection ID"=w302:refnum<k5>)  [unwired: 4 in]
              n157 = local write "Steps per pulse 3"(w338) -> ()
              n158 = call "controlRealTimeInChangePerPulse.vi"("Set"=FALSE, "error in"=w318, "axis in"=w310, "connection ID"=w302) -> ("error out"=w319:errorcluster, "Change out"=w337:i32, "axis out"=w311:u8, "connection ID"=w303:refnum<k5>)  [unwired: 4 in]
              n159 = local write "Change per pulse 3"(w337) -> ()
              n160 = call "controlRealtimeInputMove.vi"("Set"=FALSE, "error in"=w319, "axis in"=w311, "connection ID"=w303) -> ("error out"=w320:errorcluster, "move out"=w336:bool, "axis out"=w312:u8, "connection ID"=w304:refnum<k5>)  [unwired: 4 in]
              n161 = local write "RT in move Signal 3"(w336) -> ()
              n162 = local write "RT in move 3"(w336) -> ()
              n163 = call "controlAQuadBInResolution.vi"("Set"=FALSE, "error in"=w320, "axis in"=w312, "connection ID"=w304) -> ("error out"=w321:errorcluster, "Resolution out"=w335:i32, "axis out"=w313:u8, "connection ID"=w305:refnum<k5>)  [unwired: 3 in]
              n164 = local write "AquadB in res 3"(w335) -> ()
              n165 = call "controlAQuadBOut.vi"("Set"=FALSE, "error in"=w321, "axis in"=w313, "connection ID"=w305) -> ("error out"=w322:errorcluster, "ABout out"=w334:bool, "axis out"=w314:u8, "connection ID"=w306:refnum<k5>)  [unwired: 4 in]
              n166 = local write "AquadB out 3"(w334) -> ()
              n167 = call "controlAQuadBOutClock.vi"("Set"=FALSE, "error in"=w322, "axis in"=w314, "connection ID"=w306) -> ("error out"=w323:errorcluster, "clock out"=w333:i32, "axis out"=w315:u8, "connection ID"=w307:refnum<k5>)  [unwired: 4 in]
              n168 = local write "AqaudB clock 3"(w333) -> ()
              n169 = call "controlAQuadBOutResolution.vi"("Set"=FALSE, "error in"=w323, "axis in"=w315, "connection ID"=w307) -> ("ABoutRes out"=w332:i32)  [unwired: 4 in, 3 out]
              n170 = local write "AquadB Resolution 3"(w332) -> ()
            }
          }
        }
        frame #1 {
          # "Main Loop"
          n171 = while {
            tunnel: w342 -> [w343]
            stop <- "stop" stop-if-true
            n172 = case shown="\"Navigation\", Par défaut" "Tab Control" {
              tunnel: w343 -> [w346 w941 w1329]
              frame "Navigation", Default {
                n173 = stacked-sequence {
                  tunnel: w346 -> [w347 w561 w751]
                  frame #0 {
                    w353 = u8 0 items=["1", "2", "3"] ("axis in")
                    # "update Axis 1"
                    n174 = event shown="[16] \"find ref\": Valeur changée" {
                      selector: _ -> [_ _ _ _ _ _ _ _ _ _ _ _ _ _ _ _ _ _ _]
                      dyn-events: _ -> [_ _ _ _ _ _ _ _ _ _ _ _ _ _ _ _ _ _ _]
                      timeout: 10 -> [_ _ _ _ _ _ _ _ _ _ _ _ _ _ _ _ _ _ _]
                      tunnel: w353 -> [w359 w370 _ w388 w397 w403 w412 w419 w424 w429 w440 w452 _ w464 w472 w483 w493 w514 w546]
                      tunnel: [w356 w366 w376 w385 w395 w402 w410 w417 w422 w427 w438 w449 _ w461 w469 w479 w492 w512 w529] -> w351
                      tunnel: w347 -> [w360 w371 w379 w389 w398 w404 w413 w420 w425 w430 w441 w453 _ w465 w473 w484 w494 w516 w547]
                      event "Amplitude [V]": Value Change {
                        n175 = event-data() -> ()  [unwired: 1 in, 1 out]
                        n176 = call "controlAmplitude.vi"("Set"=TRUE, "amplitude [V] in"="Amplitude [V]", "axis in"=w359, "connection ID"=w360) -> ("error out"=w361:errorcluster, "axis out"=w363:u8, "connection ID"=w364:refnum<k5>)  [unwired: 4 in, 1 out]
                        n177 = call "controlAmplitude.vi"("Set"=FALSE, "error in"=w361, "axis in"=w363, "connection ID"=w364) -> ("error out"=w356:errorcluster, "amplitude [V] out"=w357:dbl)  [unwired: 4 in, 2 out]
                        n178 = local write "Amplitude [V]"(w357) -> ()
                      }
                      event "Output": Value Change {
                        n179 = event-data() -> ()  [unwired: 1 in, 1 out]
                        n180 = call "controlOutput.vi"("Set"=TRUE, "enable output in"="Output", "axis in"=w370, "connection ID"=w371) -> ("error out"=w367:errorcluster, "axis out"=w372:u8, "connection ID"=w373:refnum<k5>)  [unwired: 4 in, 1 out]
                        n181 = call "controlOutput.vi"("Set"=FALSE, "error in"=w367, "axis in"=w372, "connection ID"=w373) -> ("error out"=w366:errorcluster, "enable output out"=→"Output Status 1":bool)  [unwired: 4 in, 2 out]
                      }
                      event "Frequency [Hz]": Value Change {
                        n182 = event-data() -> ()  [unwired: 1 in, 1 out]
                        n183 = call "controlFrequenzy.vi"("Set"=TRUE, "Frequenzy [Hz] in"="Frequency [Hz]", "connection ID"=w379) -> ("error out"=w380:errorcluster, "axis out"=w381:u8, "connection ID"=w384:refnum<k5>)  [unwired: 5 in, 1 out]
                        n184 = call "controlFrequenzy.vi"("Set"=FALSE, "error in"=w380, "axis in"=w381, "connection ID"=w384) -> ("error out"=w376:errorcluster, "Frequenzy [Hz] out"=w377:dbl)  [unwired: 4 in, 2 out]
                        n185 = local write "Frequency [Hz]"(w377) -> ()
                      }
                      event "Move": Value Change {
                        n186 = event-data() -> ()  [unwired: 1 in, 1 out]
                        n187 = call "controlMove.vi"("Set"=TRUE, "control move in"="Move", "axis in"=w388, "connection ID"=w389) -> ("error out"=w390:errorcluster, "axis out"=w391:u8, "connection ID"=w394:refnum<k5>)  [unwired: 4 in, 1 out]
                        n188 = call "controlMove.vi"("Set"=FALSE, "error in"=w390, "axis in"=w391, "connection ID"=w394) -> ("error out"=w385:errorcluster, "controll move out"=→"move out":bool)  [unwired: 4 in, 2 out]
                      }
                      event "EoT 1": Value Change {
                        n189 = event-data() -> ()  [unwired: 1 in, 1 out]
                        n190 = call "controlEotOutputDeactive.vi"("Set"=TRUE, "enable EOT in"="EoT 1", "axis in"=w397, "connection ID"=w398) -> ("error out"=w395:errorcluster)  [unwired: 4 in, 3 out]
                      }
                      event "Target Position 1": Value Change {
                        n191 = event-data() -> ()  [unwired: 1 in, 1 out]
                        n192 = call "controlTargetPosition.vi"("Set"=TRUE, "Target Position in"="Target Position 1", "axis in"=w403, "connection ID"=w404) -> ("error out"=w406:errorcluster, "axis out"=w407:u8, "connection ID"=w408:refnum<k5>)  [unwired: 4 in, 1 out]
                        n193 = call "controlTargetPosition.vi"("Set"=FALSE, "error in"=w406, "axis in"=w407, "connection ID"=w408) -> ("error out"=w402:errorcluster, "Target Position out"=w400:dbl)  [unwired: 4 in, 2 out]
                        n194 = local write "Target Position 1"(w400) -> ()
                      }
                      event "Axis 1": Value Change {
                        n195 = event-data() -> ()  [unwired: 1 in, 1 out]
                        n196 = case shown="Vrai" "Axis 1" {
                          tunnel: [_ w416] -> w410
                          tunnel: w413 -> [_ w415]
                          tunnel: w412 -> [_ w414]
                          frame False {
                          }
                          frame True {
                            n197 = call "setReset.vi"("axis in"=w414, "connection ID"=w415) -> ("error out"=w416:errorcluster)  [unwired: 7 in, 2 out]
                          }
                        }
                      }
                      event "Single Step Left": Value Change {
                        n198 = event-data() -> ()  [unwired: 1 in, 1 out]
                        n199 = call "setNSteps.vi"("FWD"=TRUE, "setnSteps in"="Number of steps 1", "axis in"=w419, "connection ID"=w420) -> ("error out"=w417:errorcluster)  [unwired: 4 in, 3 out]
                      }
                      event "Single Step Right": Value Change {
                        n200 = event-data() -> ()  [unwired: 1 in, 1 out]
                        n201 = local read "Number of steps 1"() -> (w423:i32)
                        n202 = call "setNSteps.vi"("FWD"=FALSE, "setnSteps in"=w423, "axis in"=w424, "connection ID"=w425) -> ("error out"=w422:errorcluster)  [unwired: 4 in, 3 out]
                      }
                      event "Endless Left": Value Change {
                        n203 = event-data() -> ()  [unwired: 1 in, 1 out]
                        n204 = call "controlContinousFwd.vi"("Set"=TRUE, "continous FWD in"=FALSE, "axis in"=w429, "connection ID"=w430) -> ("error out"=w431:errorcluster, "axis out"=w435:u8, "connection ID"=w436:refnum<k5>)  [unwired: 4 in, 1 out]
                        n205 = call "controlContinousBkwd.vi"("Set"=TRUE, "error in"=w431, "continous BWD in"="Endless Left", "axis in"=w435, "connection ID"=w436) -> ("error out"=w427:errorcluster)  [unwired: 3 in, 3 out]
                        n206 = local write "Continuous Forward"(FALSE) -> ()
                      }
                      event "Continuous Forward": Value Change {
                        n207 = event-data() -> ()  [unwired: 1 in, 1 out]
                        n208 = call "controlContinousBkwd.vi"("Set"=TRUE, "continous BWD in"=FALSE, "axis in"=w440, "connection ID"=w441) -> ("error out"=w442:errorcluster, "axis out"=w446:u8, "connection ID"=w447:refnum<k5>)  [unwired: 4 in, 1 out]
                        n209 = call "controlContinousFwd.vi"("Set"=TRUE, "error in"=w442, "continous FWD in"="Continuous Forward", "axis in"=w446, "connection ID"=w447) -> ("error out"=w438:errorcluster)  [unwired: 3 in, 3 out]
                        n210 = local write "Endless Left"(FALSE) -> ()
                      }
                      event "Fixed DC 1": Value Change {
                        n211 = event-data() -> ()  [unwired: 1 in, 1 out]
                        n212 = call "controlFixOutputVoltage.vi"("Set"=TRUE, "Fixed Output Voltage in"="Fixed DC 1", "axis in"=w452, "connection ID"=w453) -> ("error out"=w454:errorcluster, "axis out"=w455:u8, "connection ID"=w456:refnum<k5>)  [unwired: 4 in, 1 out]
                        n213 = call "controlFixOutputVoltage.vi"("Set"=FALSE, "error in"=w454, "axis in"=w455, "connection ID"=w456) -> ("error out"=w449:errorcluster, "Fixed Output Voltage out"=w450:dbl)  [unwired: 4 in, 2 out]
                        n214 = local write "Fixed DC 1"(w450) -> ()
                      }
                      event "Reset Error": Value Change {
                        n215 = event-data() -> ()  [unwired: 1 in, 1 out]
                        n216 = local write "Error Message"("" ("Error Message")) -> ()
                        n217 = local write "Error"(FALSE ("Error")) -> ()
                      }
                      event "Positioner": Value Change {
                        n218 = event-data() -> ()  [unwired: 1 in, 1 out]
                        n219 = property on="Positioner" class="MDér (strict)"() -> ("RingText.Text"=w463:string)  [unwired: 2 in, 2 out]
                        n220 = call "controlActorSelection.vi"("Positioner in"=w463, "axis in"=w464, "connection ID"=w465) -> ("error out"=w466:errorcluster, "axis out"=w467:u8, "connection ID"=w468:refnum<k5>)  [unwired: 6 in]
                        n221 = call "getActorType.vi"("error in"=w466, "axis in"=w467, "connection ID"=w468) -> ("error out"=w461:errorcluster, "Actor Type"=w462:dbl)  [unwired: 5 in, 2 out]
                        n222 = local write "actor type"(w462) -> ()
                      }
                      event "Target Range 1": Value Change {
                        n223 = event-data() -> ()  [unwired: 1 in, 1 out]
                        n224 = call "controlTargetRange.vi"("Set"=TRUE, "Target Range in"="Target Range 1", "axis in"=w472, "connection ID"=w473) -> ("error out"=w475:errorcluster, "axis out"=w476:u8, "connection ID"=w477:refnum<k5>)  [unwired: 4 in, 1 out]
                        n225 = call "controlTargetRange.vi"("Set"=FALSE, "error in"=w475, "axis in"=w476, "connection ID"=w477) -> ("error out"=w469:errorcluster, "Target Range out"=w470:dbl)  [unwired: 4 in, 2 out]
                        n226 = local write "Target Range 1"(w470) -> ()
                      }
                      event "auto Reset 1": Value Change {
                        n227 = event-data() -> ()  [unwired: 1 in, 1 out]
                        n228 = call "controlAutoReset.vi"("Set"=TRUE, "auto reset in"="auto Reset 1", "axis in"=w483, "connection ID"=w484) -> ("error out"=w480:errorcluster, "axis out"=w487:u8, "connection ID"=w486:refnum<k5>)  [unwired: 4 in, 1 out]
                        n229 = call "controlAutoReset.vi"("Set"=FALSE, "error in"=w480, "axis in"=w487, "connection ID"=w486) -> ("error out"=w479:errorcluster, "auto reset out"=w481:bool)  [unwired: 4 in, 2 out]
                        n230 = local write "auto Reset 1"(w481) -> ()
                      }
                      event "find ref": Value Change {
                        n231 = event-data() -> ("NewVal"=w491:bool)  [unwired: 1 in, 5 out]
                        n232 = case shown="Vrai" w491 {
                          tunnel: w494 -> [_ w501]
                          tunnel: w493 -> [_ _]
                          tunnel: [_ w502] -> w492
                          tunnel: [_ FALSE ("Set")] -> w490
                          tunnel: "Find" -> [_ w496]
                          frame False {
                          }
                          frame True {
                            n233 = case shown="Vrai" w496 {
                              tunnel: w501 -> [w504 w508]
                              tunnel: "axis in" -> [_ w507]
                              tunnel: [_ w506] -> w499
                              tunnel: [w504 w505] -> w498
                              frame False {
                              }
                              frame True {
                                n234 = call "moveReference.vi"("axis in"=w507, "connection ID"=w508) -> ("error out"=w506:errorcluster, "connection ID"=w505:refnum<k5>)  [unwired: 6 in, 2 out]
                              }
                            }
                            n235 = while {
                              tunnel: [w510] -> w500
                              tunnel: w499 -> [w510]
                              stop <- "stop 2" stop-if-true
                              n236 = Wait (ms)(milliseconds to wait=u32 200 ("attente (ms)")) -> ()  [unwired: 1 out]
                            }
                            n237 = call "getStatusReference.vi"("error in"=w500, "axis in"="axis in", "connection ID"=w498) -> ("error out"=w502:errorcluster, "status reference out"=→"status reference out":bool)  [unwired: 5 in, 2 out]
                          }
                        }
                        n238 = local write "find ref"(w490) -> ()
                      }
                      event "Reference Auto Update 1": Value Change {
                        n239 = event-data() -> ()  [unwired: 1 in, 1 out]
                        n240 = call "controlReferenceAutoUpdate.vi"("Set"=TRUE, "ref auto up in"="Reference Auto Update 1", "axis in"=w514, "connection ID"=w516) -> ("error out"=w521:errorcluster, "axis out"=w520:u8, "connection ID"=w519:refnum<k5>)  [unwired: 4 in, 1 out]
                        n241 = call "controlReferenceAutoUpdate.vi"("Set"=FALSE, "error in"=w521, "axis in"=w520, "connection ID"=w519) -> ("error out"=w512:errorcluster, "ref auto up out"=w513:bool)  [unwired: 4 in, 2 out]
                        n242 = local write "Reference Auto Update 1"(w513) -> ()
                      }
                      event Timeout {
                        n243 = event-data() -> ()  [unwired: 1 in, 1 out]
                        n244 = call "getPosition.vi"("axis in"=w546, "connection ID"=w547) -> ("error out"=w538:errorcluster, "position out"=→"Position":dbl, "axis out"=w559:u8, "connection ID"=w560:refnum<k5>)  [unwired: 6 in]
                        n245 = call "getReferencePosition.vi"("error in"=w538, "axis in"=w559, "connection ID"=w560) -> ("error out"=w524:errorcluster, "Reference position out"=→"Reference":dbl, "axis out"=w558:u8, "connection ID"=w525:refnum<k5>)  [unwired: 5 in]
                        n246 = call "getOutputVoltage.vi"("error in"=w524, "connection ID"=w525) -> ("error out"=w522:errorcluster, "Voltage (mv)"=→"Voltage (mv)":i64)  [unwired: 6 in, 2 out]
                        n247 = call "getStatusConnected.vi"("error in"=w522, "axis in"=w558, "connection ID"=w525) -> ("error out"=w537:errorcluster, "Status Connected out"=→"Connected":bool, "axis out"=w556:u8, "connection ID"=w557:refnum<k5>)  [unwired: 5 in]
                        n248 = call "getStatusMoving.vi"("error in"=w537, "axis in"=w556, "connection ID"=w557) -> ("error out"=w536:errorcluster, "status moving out"=→"MoveSignal":bool, "axis out"=w554:u8, "connection ID"=w555:refnum<k5>)  [unwired: 5 in]
                        n249 = call "getStatusReference.vi"("error in"=w536, "axis in"=w554, "connection ID"=w555) -> ("error out"=w535:errorcluster, "status reference out"=→"ReferenceSignal":bool, "axis out"=w552:u8, "connection ID"=w553:refnum<k5>)  [unwired: 5 in]
                        n250 = call "getStatusEotBkwd.vi"("error in"=w535, "axis in"=w552, "connection ID"=w553) -> ("error out"=w534:errorcluster, "Get Stus EOT BKWD out"=→"EotLeftDetected1":bool, "axis out"=w550:u8, "connection ID"=w551:refnum<k5>)  [unwired: 5 in]
                        n251 = call "getStatusEotFwd.vi"("error in"=w534, "axis in"=w550, "connection ID"=w551) -> ("error out"=w533:errorcluster, "Status EOT FWD out"=→"EotrightDetected1":bool, "axis out"=w548:u8, "connection ID"=w549:refnum<k5>)  [unwired: 5 in]
                        n252 = call "getStatusTargetRange.vi"("error in"=w533, "axis in"=w548, "connection ID"=w549) -> ("error out"=w530:errorcluster, "Status Target Range out"=→"in target range1":bool, "axis out"=w531:u8, "connection ID"=w532:refnum<k5>)  [unwired: 5 in]
                        n253 = call "controlMove.vi"("Set"=FALSE, "error in"=w530, "axis in"=w531, "connection ID"=w532) -> ("error out"=w529:errorcluster, "controll move out"=w527:bool)  [unwired: 4 in, 2 out]
                        n254 = local write "Move"(w527) -> ()
                        n255 = local write "move out"(w527) -> ()
                      }
                    }
                    n256 = Unbundle(w351) -> ("code"=w349:i32, "source"=w350:string)  [unwired: 1 out]
                    n257 = Not Equal To 0?(x=w349) -> (x != 0?=w348:bool)
                    n258 = case shown="Faux" w348 {
                      selector: w348 -> [_ w354]
                      tunnel: w350 -> [_ w355]
                      frame False {
                      }
                      frame True {
                        "Error Message" <- w355
                        "Error" <- w354
                      }
                    }
                  }
                  frame #1 {
                    w567 = u8 1 items=["1", "2", "3"] ("axis in")
                    # "update Axis 2"
                    n259 = event shown="[17] Timeout" {
                      selector: _ -> [_ _ _ _ _ _ _ _ _ _ _ _ _ _ _ _ _ _]
                      dyn-events: _ -> [_ _ _ _ _ _ _ _ _ _ _ _ _ _ _ _ _ _]
                      timeout: 10 -> [_ _ _ _ _ _ _ _ _ _ _ _ _ _ _ _ _ _]
                      tunnel: w567 -> [w576 w587 w595 w605 w613 w623 w626 w635 w640 w649 w660 w669 _ w681 w690 w702 w712 w731]
                      tunnel: [w570 w582 w590 w600 w610 w618 w625 w633 w637 w642 w654 w666 _ w676 w686 w694 w704 w719] -> w564
                      tunnel: w561 -> [w579 w589 w599 w609 w614 w624 w627 w636 w641 w651 w662 w673 _ w683 w693 w703 w713 w750]
                      event "amplitude [V] 2": Value Change {
                        n260 = event-data() -> ()  [unwired: 1 in, 1 out]
                        n261 = call "controlAmplitude.vi"("Set"=TRUE, "amplitude [V] in"="amplitude [V] 2", "axis in"=w576, "connection ID"=w579) -> ("error out"=w571:errorcluster, "axis out"=w575:u8, "connection ID"=w577:refnum<k5>)  [unwired: 4 in, 1 out]
                        n262 = call "controlAmplitude.vi"("Set"=FALSE, "error in"=w571, "axis in"=w575, "connection ID"=w577) -> ("error out"=w570:errorcluster, "amplitude [V] out"=w572:dbl)  [unwired: 4 in, 2 out]
                        n263 = local write "amplitude [V] 2"(w572) -> ()
                      }
                      event "Output 2": Value Change {
                        n264 = event-data() -> ()  [unwired: 1 in, 1 out]
                        n265 = call "controlOutput.vi"("Set"=TRUE, "enable output in"="Output 2", "axis in"=w587, "connection ID"=w589) -> ("error out"=w580:errorcluster, "axis out"=w583:u8, "connection ID"=w584:refnum<k5>)  [unwired: 4 in, 1 out]
                        n266 = call "controlOutput.vi"("Set"=FALSE, "error in"=w580, "axis in"=w583, "connection ID"=w584) -> ("error out"=w582:errorcluster, "enable output out"=→"Output Status 2":bool)  [unwired: 4 in, 2 out]
                      }
                      event "frequency [Hz] 2": Value Change {
                        n267 = event-data() -> ()  [unwired: 1 in, 1 out]
                        n268 = call "controlFrequenzy.vi"("Set"=TRUE, "Frequenzy [Hz] in"="frequency [Hz] 2", "axis in"=w595, "connection ID"=w599) -> ("error out"=w591:errorcluster, "axis out"=w594:u8, "connection ID"=w598:refnum<k5>)  [unwired: 4 in, 1 out]
                        n269 = call "controlFrequenzy.vi"("Set"=FALSE, "error in"=w591, "axis in"=w594, "connection ID"=w598) -> ("error out"=w590:errorcluster, "Frequenzy [Hz] out"=w593:dbl)  [unwired: 4 in, 2 out]
                        n270 = local write "frequency [Hz] 2"(w593) -> ()
                      }
                      event "Move 2": Value Change {
                        n271 = event-data() -> ()  [unwired: 1 in, 1 out]
                        n272 = call "controlMove.vi"("Set"=TRUE, "control move in"="Move 2", "axis in"=w605, "connection ID"=w609) -> ("error out"=w601:errorcluster, "axis out"=w604:u8, "connection ID"=w608:refnum<k5>)  [unwired: 4 in, 1 out]
                        n273 = call "controlMove.vi"("Set"=FALSE, "error in"=w601, "axis in"=w604, "connection ID"=w608) -> ("error out"=w600:errorcluster, "controll move out"=→"move out 2":bool)  [unwired: 4 in, 2 out]
                      }
                      event "EoT 2": Value Change {
                        n274 = event-data() -> ()  [unwired: 1 in, 1 out]
                        n275 = call "controlEotOutputDeactive.vi"("Set"=TRUE, "enable EOT in"="EoT 2", "axis in"=w613, "connection ID"=w614) -> ("error out"=w610:errorcluster)  [unwired: 4 in, 3 out]
                      }
                      event "Target position 2": Value Change {
                        n276 = event-data() -> ()  [unwired: 1 in, 1 out]
                        n277 = call "controlTargetPosition.vi"("Set"=TRUE, "Target Position in"="Target position 2", "axis in"=w623, "connection ID"=w624) -> ("error out"=w619:errorcluster, "axis out"=w620:u8, "connection ID"=w621:refnum<k5>)  [unwired: 4 in, 1 out]
                        n278 = call "controlTargetPosition.vi"("Set"=FALSE, "error in"=w619, "axis in"=w620, "connection ID"=w621) -> ("error out"=w618:errorcluster, "Target Position out"=w616:dbl)  [unwired: 4 in, 2 out]
                        n279 = local write "Target position 2"(w616) -> ()
                      }
                      event "Axis 2": Value Change {
                        n280 = event-data() -> ()  [unwired: 1 in, 1 out]
                        n281 = case shown="Vrai" "Axis 2" {
                          tunnel: w627 -> [_ w631]
                          tunnel: w626 -> [_ w630]
                          tunnel: [_ w629] -> w625
                          frame False {
                          }
                          frame True {
                            n282 = call "setReset.vi"("axis in"=w630, "connection ID"=w631) -> ("error out"=w629:errorcluster)  [unwired: 7 in, 2 out]
                          }
                        }
                      }
                      event "Single Step Left 2": Value Change {
                        n283 = event-data() -> ()  [unwired: 1 in, 1 out]
                        n284 = call "setNSteps.vi"("FWD"=TRUE, "setnSteps in"="Number of steps 2", "axis in"=w635, "connection ID"=w636) -> ("error out"=w633:errorcluster)  [unwired: 4 in, 3 out]
                      }
                      event "Single Step Right 2": Value Change {
                        n285 = event-data() -> ()  [unwired: 1 in, 1 out]
                        n286 = local read "Number of steps 2"() -> (w639:i32)
                        n287 = call "setNSteps.vi"("FWD"=FALSE, "setnSteps in"=w639, "axis in"=w640, "connection ID"=w641) -> ("error out"=w637:errorcluster)  [unwired: 4 in, 3 out]
                      }
                      event "Endless Left 2": Value Change {
                        n288 = event-data() -> ()  [unwired: 1 in, 1 out]
                        n289 = call "controlContinousFwd.vi"("Set"=TRUE, "continous FWD in"=FALSE, "axis in"=w649, "connection ID"=w651) -> ("error out"=w643:errorcluster, "axis out"=w648:u8, "connection ID"=w650:refnum<k5>)  [unwired: 4 in, 1 out]
                        n290 = call "controlContinousBkwd.vi"("Set"=TRUE, "error in"=w643, "continous BWD in"="Endless Left 2", "axis in"=w648, "connection ID"=w650) -> ("error out"=w642:errorcluster)  [unwired: 3 in, 3 out]
                        n291 = local write "Continuous Forward"(FALSE) -> ()
                      }
                      event "Continuous Forward": Value Change {
                        n292 = event-data() -> ()  [unwired: 1 in, 1 out]
                        n293 = call "controlContinousBkwd.vi"("Set"=TRUE, "continous BWD in"=FALSE, "axis in"=w660, "connection ID"=w662) -> ("error out"=w655:errorcluster, "axis out"=w659:u8, "connection ID"=w661:refnum<k5>)  [unwired: 4 in, 1 out]
                        n294 = call "controlContinousFwd.vi"("Set"=TRUE, "error in"=w655, "continous FWD in"="Continuous Forward", "axis in"=w659, "connection ID"=w661) -> ("error out"=w654:errorcluster)  [unwired: 3 in, 3 out]
                        n295 = local write "Endless Left 2"(FALSE ("Endless Left 2")) -> ()
                      }
                      event "Fixed DC 2": Value Change {
                        n296 = event-data() -> ()  [unwired: 1 in, 1 out]
                        n297 = call "controlFixOutputVoltage.vi"("Set"=TRUE, "Fixed Output Voltage in"="Fixed DC 2", "axis in"=w669, "connection ID"=w673) -> ("error out"=w667:errorcluster, "axis out"=w668:u8, "connection ID"=w670:refnum<k5>)  [unwired: 4 in, 1 out]
                        n298 = call "controlFixOutputVoltage.vi"("Set"=FALSE, "error in"=w667, "axis in"=w668, "connection ID"=w670) -> ("error out"=w666:errorcluster, "Fixed Output Voltage out"=w664:dbl)  [unwired: 4 in, 2 out]
                        n299 = local write "Fixed DC 2"(w664) -> ()
                      }
                      event "Reset Error 2": Value Change {
                        n300 = event-data() -> ()  [unwired: 1 in, 1 out]
                        n301 = local write "Error Message 2"("" ("Error Message 2")) -> ()
                        n302 = local write "Error 2"(FALSE ("Error 2")) -> ()
                      }
                      event "Positioner 2": Value Change {
                        n303 = event-data() -> ()  [unwired: 1 in, 1 out]
                        n304 = property on="Positioner 2" class="MDér (strict)"() -> ("RingText.Text"=w682:string)  [unwired: 2 in, 2 out]
                        n305 = call "controlActorSelection.vi"("Positioner in"=w682, "axis in"=w681, "connection ID"=w683) -> ("error out"=w677:errorcluster, "axis out"=w679:u8, "connection ID"=w680:refnum<k5>)  [unwired: 6 in]
                        n306 = call "getActorType.vi"("error in"=w677, "axis in"=w679, "connection ID"=w680) -> ("error out"=w676:errorcluster, "Actor Type"=w678:dbl)  [unwired: 5 in, 2 out]
                        n307 = local write "actor type 2"(w678) -> ()
                      }
                      event "Target Range 2": Value Change {
                        n308 = event-data() -> ()  [unwired: 1 in, 1 out]
                        n309 = call "controlTargetRange.vi"("Set"=TRUE, "Target Range in"="Target Range 2", "axis in"=w690, "connection ID"=w693) -> ("error out"=w687:errorcluster, "axis out"=w688:u8, "connection ID"=w689:refnum<k5>)  [unwired: 4 in, 1 out]
                        n310 = call "controlTargetRange.vi"("Set"=FALSE, "error in"=w687, "axis in"=w688, "connection ID"=w689) -> ("error out"=w686:errorcluster, "Target Range out"=w685:dbl)  [unwired: 4 in, 2 out]
                        n311 = local write "Target Range 2"(w685) -> ()
                      }
                      event "auto Reset 2": Value Change {
                        n312 = event-data() -> ()  [unwired: 1 in, 1 out]
                        n313 = call "controlAutoReset.vi"("Set"=TRUE, "auto reset in"="auto Reset 2", "axis in"=w702, "connection ID"=w703) -> ("error out"=w695:errorcluster, "axis out"=w699:u8, "connection ID"=w700:refnum<k5>)  [unwired: 4 in, 1 out]
                        n314 = call "controlAutoReset.vi"("Set"=FALSE, "error in"=w695, "axis in"=w699, "connection ID"=w700) -> ("error out"=w694:errorcluster, "auto reset out"=w696:bool)  [unwired: 4 in, 2 out]
                        n315 = local write "auto Reset 2"(w696) -> ()
                      }
                      event "Reference Auto Update 2": Value Change {
                        n316 = event-data() -> ()  [unwired: 1 in, 1 out]
                        n317 = call "controlReferenceAutoUpdate.vi"("Set"=TRUE, "ref auto up in"="Reference Auto Update 2", "axis in"=w712, "connection ID"=w713) -> ("error out"=w707:errorcluster, "axis out"=w708:u8, "connection ID"=w709:refnum<k5>)  [unwired: 4 in, 1 out]
                        n318 = call "controlReferenceAutoUpdate.vi"("Set"=FALSE, "error in"=w707, "axis in"=w708, "connection ID"=w709) -> ("error out"=w704:errorcluster, "ref auto up out"=w705:bool)  [unwired: 4 in, 2 out]
                        n319 = local write "Reference Auto Update 2"(w705) -> ()
                      }
                      event Timeout {
                        n320 = event-data() -> ()  [unwired: 1 in, 1 out]
                        n321 = call "getPosition.vi"("axis in"=w731, "connection ID"=w750) -> ("error out"=w727:errorcluster, "position out"=→"Position 2":dbl, "axis out"=w747:u8, "connection ID"=w748:refnum<k5>)  [unwired: 6 in]
                        n322 = call "getReferencePosition.vi"("error in"=w727, "axis in"=w747, "connection ID"=w748) -> ("error out"=w726:errorcluster, "Reference position out"=→"Reference 2":dbl, "axis out"=w744:u8, "connection ID"=w745:refnum<k5>)  [unwired: 5 in]
                        n323 = call "getStatusConnected.vi"("error in"=w726, "axis in"=w744, "connection ID"=w745) -> ("error out"=w725:errorcluster, "Status Connected out"=→"Connected 2":bool, "axis out"=w741:u8, "connection ID"=w742:refnum<k5>)  [unwired: 5 in]
                        n324 = call "getStatusMoving.vi"("error in"=w725, "axis in"=w741, "connection ID"=w742) -> ("error out"=w724:errorcluster, "status moving out"=→"MoveSignal 2":bool, "axis out"=w738:u8, "connection ID"=w739:refnum<k5>)  [unwired: 5 in]
                        n325 = call "getStatusReference.vi"("error in"=w724, "axis in"=w738, "connection ID"=w739) -> ("error out"=w723:errorcluster, "status reference out"=→"ReferenceSignal 2":bool, "axis out"=w735:u8, "connection ID"=w736:refnum<k5>)  [unwired: 5 in]
                        n326 = call "getStatusEotBkwd.vi"("error in"=w723, "axis in"=w735, "connection ID"=w736) -> ("error out"=w722:errorcluster, "Get Stus EOT BKWD out"=→"EotLeftDetected2":bool, "axis out"=w733:u8, "connection ID"=w734:refnum<k5>)  [unwired: 5 in]
                        n327 = call "getStatusEotFwd.vi"("error in"=w722, "axis in"=w733, "connection ID"=w734) -> ("error out"=w721:errorcluster, "Status EOT FWD out"=→"EotrightDetected2":bool, "axis out"=w728:u8, "connection ID"=w729:refnum<k5>)  [unwired: 5 in]
                        n328 = call "getStatusTargetRange.vi"("error in"=w721, "axis in"=w728, "connection ID"=w729) -> ("error out"=w720:errorcluster, "Status Target Range out"=→"in target range2":bool, "axis out"=w716:u8, "connection ID"=w717:refnum<k5>)  [unwired: 5 in]
                        n329 = call "controlMove.vi"("Set"=FALSE, "error in"=w720, "axis in"=w716, "connection ID"=w717) -> ("error out"=w719:errorcluster, "controll move out"=w715:bool)  [unwired: 4 in, 2 out]
                        n330 = local write "move out 2"(w715) -> ()
                        n331 = local write "Move 2"(w715) -> ()
                      }
                    }
                    n332 = Unbundle(w564) -> ("code"=w563:i32, "source"=w565:string)  [unwired: 1 out]
                    n333 = Not Equal To 0?(x=w563) -> (x != 0?=w562:bool)
                    n334 = case shown="Faux" w562 {
                      selector: w562 -> [_ w568]
                      tunnel: w565 -> [_ w569]
                      frame False {
                      }
                      frame True {
                        "Error Message 2" <- w569
                        "Error 2" <- w568
                      }
                    }
                  }
                  frame #2 {
                    w757 = u8 2 items=["1", "2", "3"] ("axis in")
                    # "update Axis 3"
                    n335 = event shown="[15] \"auto Reset 3\": Valeur changée" {
                      selector: _ -> [_ _ _ _ _ _ _ _ _ _ _ _ _ _ _ _ _ _]
                      dyn-events: _ -> [_ _ _ _ _ _ _ _ _ _ _ _ _ _ _ _ _ _]
                      timeout: 10 -> [_ _ _ _ _ _ _ _ _ _ _ _ _ _ _ _ _ _]
                      tunnel: w757 -> [w763 w774 w783 w793 w802 w808 w817 w824 w829 w834 w845 w856 _ w869 w877 w888 w896 w924]
                      tunnel: [w760 w770 w780 w790 w800 w806 w815 w822 w827 w832 w843 w854 _ w867 w874 w884 w894 w906] -> w754
                      tunnel: w751 -> [w764 w775 w784 w794 w803 w809 w818 w825 w830 w835 w846 w858 _ w870 w878 w889 w898 w925]
                      event "amplitude [V] 3": Value Change {
                        n336 = event-data() -> ()  [unwired: 1 in, 1 out]
                        n337 = call "controlAmplitude.vi"("Set"=TRUE, "amplitude [V] in"="amplitude [V] 3", "axis in"=w763, "connection ID"=w764) -> ("error out"=w765:errorcluster, "axis out"=w767:u8, "connection ID"=w768:refnum<k5>)  [unwired: 4 in, 1 out]
                        n338 = call "controlAmplitude.vi"("Set"=FALSE, "error in"=w765, "axis in"=w767, "connection ID"=w768) -> ("error out"=w760:errorcluster, "amplitude [V] out"=w761:dbl)  [unwired: 4 in, 2 out]
                        n339 = local write "amplitude [V] 3"(w761) -> ()
                      }
                      event "Output 3": Value Change {
                        n340 = event-data() -> ()  [unwired: 1 in, 1 out]
                        n341 = call "controlOutput.vi"("Set"=TRUE, "enable output in"="Output 3", "axis in"=w774, "connection ID"=w775) -> ("error out"=w771:errorcluster, "axis out"=w776:u8, "connection ID"=w777:refnum<k5>)  [unwired: 4 in, 1 out]
                        n342 = call "controlOutput.vi"("Set"=FALSE, "error in"=w771, "axis in"=w776, "connection ID"=w777) -> ("error out"=w770:errorcluster, "enable output out"=→"Output Satus 3":bool)  [unwired: 4 in, 2 out]
                      }
                      event "frequency [Hz] 3": Value Change {
                        n343 = event-data() -> ()  [unwired: 1 in, 1 out]
                        n344 = call "controlFrequenzy.vi"("Set"=TRUE, "Frequenzy [Hz] in"="frequency [Hz] 3", "axis in"=w783, "connection ID"=w784) -> ("error out"=w785:errorcluster, "axis out"=w786:u8, "connection ID"=w789:refnum<k5>)  [unwired: 4 in, 1 out]
                        n345 = call "controlFrequenzy.vi"("Set"=FALSE, "error in"=w785, "axis in"=w786, "connection ID"=w789) -> ("error out"=w780:errorcluster, "Frequenzy [Hz] out"=w781:dbl)  [unwired: 4 in, 2 out]
                        n346 = local write "frequency [Hz] 3"(w781) -> ()
                      }
                      event "Move 3": Value Change {
                        n347 = event-data() -> ()  [unwired: 1 in, 1 out]
                        n348 = call "controlMove.vi"("Set"=TRUE, "control move in"="Move 3", "axis in"=w793, "connection ID"=w794) -> ("error out"=w795:errorcluster, "axis out"=w796:u8, "connection ID"=w799:refnum<k5>)  [unwired: 4 in, 1 out]
                        n349 = call "controlMove.vi"("Set"=FALSE, "error in"=w795, "axis in"=w796, "connection ID"=w799) -> ("error out"=w790:errorcluster, "controll move out"=→"move out 3":bool)  [unwired: 4 in, 2 out]
                      }
                      event "EoT 3": Value Change {
                        n350 = event-data() -> ()  [unwired: 1 in, 1 out]
                        n351 = call "controlEotOutputDeactive.vi"("Set"=TRUE, "enable EOT in"="EoT 3", "axis in"=w802, "connection ID"=w803) -> ("error out"=w800:errorcluster)  [unwired: 4 in, 3 out]
                      }
                      event "Target Position 3": Value Change {
                        n352 = event-data() -> ()  [unwired: 1 in, 1 out]
                        n353 = call "controlTargetPosition.vi"("Set"=TRUE, "Target Position in"="Target Position 3", "axis in"=w808, "connection ID"=w809) -> ("error out"=w811:errorcluster, "axis out"=w812:u8, "connection ID"=w813:refnum<k5>)  [unwired: 4 in, 1 out]
                        n354 = call "controlTargetPosition.vi"("Set"=FALSE, "error in"=w811, "axis in"=w812, "connection ID"=w813) -> ("error out"=w806:errorcluster, "axis out"=w807:u8)  [unwired: 4 in, 2 out]
                        n355 = local write "Target Position 3"(w807) -> ()
                      }
                      event "Axis 3": Value Change {
                        n356 = event-data() -> ()  [unwired: 1 in, 1 out]
                        n357 = case shown="Vrai" "Axis 3" {
                          tunnel: [_ w821] -> w815
                          tunnel: w818 -> [_ w820]
                          tunnel: w817 -> [_ w819]
                          frame False {
                          }
                          frame True {
                            n358 = call "setReset.vi"("axis in"=w819, "connection ID"=w820) -> ("error out"=w821:errorcluster)  [unwired: 7 in, 2 out]
                          }
                        }
                      }
                      event "Single Step Left 3": Value Change {
                        n359 = event-data() -> ()  [unwired: 1 in, 1 out]
                        n360 = call "setNSteps.vi"("FWD"=TRUE, "setnSteps in"="Number of steps 3", "axis in"=w824, "connection ID"=w825) -> ("error out"=w822:errorcluster)  [unwired: 4 in, 3 out]
                      }
                      event "Single Step Right 3": Value Change {
                        n361 = event-data() -> ()  [unwired: 1 in, 1 out]
                        n362 = local read "Number of steps 3"() -> (w828:i32)
                        n363 = call "setNSteps.vi"("FWD"=FALSE, "setnSteps in"=w828, "axis in"=w829, "connection ID"=w830) -> ("error out"=w827:errorcluster)  [unwired: 4 in, 3 out]
                      }
                      event "Endless Left 3": Value Change {
                        n364 = event-data() -> ()  [unwired: 1 in, 1 out]
                        n365 = call "controlContinousFwd.vi"("Set"=TRUE, "continous FWD in"=FALSE, "axis in"=w834, "connection ID"=w835) -> ("error out"=w836:errorcluster, "axis out"=w840:u8, "connection ID"=w841:refnum<k5>)  [unwired: 4 in, 1 out]
                        n366 = call "controlContinousBkwd.vi"("Set"=TRUE, "error in"=w836, "continous BWD in"="Endless Left 3", "axis in"=w840, "connection ID"=w841) -> ("error out"=w832:errorcluster)  [unwired: 3 in, 3 out]
                        n367 = local write "Continuous Forward"(FALSE ("Endless Right 3")) -> ()
                      }
                      event "Continuous Forward": Value Change {
                        n368 = event-data() -> ()  [unwired: 1 in, 1 out]
                        n369 = call "controlContinousBkwd.vi"("Set"=TRUE, "continous BWD in"=FALSE, "axis in"=w845, "connection ID"=w846) -> ("error out"=w847:errorcluster, "axis out"=w851:u8, "connection ID"=w852:refnum<k5>)  [unwired: 4 in, 1 out]
                        n370 = call "controlContinousFwd.vi"("Set"=TRUE, "error in"=w847, "continous FWD in"="Continuous Forward", "axis in"=w851, "connection ID"=w852) -> ("error out"=w843:errorcluster)  [unwired: 3 in, 3 out]
                        n371 = local write "Endless Left 3"(FALSE ("Endless Left 3")) -> ()
                      }
                      event "Fixed DC 3": Value Change {
                        n372 = event-data() -> ()  [unwired: 1 in, 1 out]
                        n373 = call "controlFixOutputVoltage.vi"("Set"=TRUE, "Fixed Output Voltage in"="Fixed DC 3", "axis in"=w856, "connection ID"=w858) -> ("error out"=w859:errorcluster, "axis out"=w860:u8, "connection ID"=w861:refnum<k5>)  [unwired: 4 in, 1 out]
                        n374 = call "controlFixOutputVoltage.vi"("Set"=FALSE, "error in"=w859, "axis in"=w860, "connection ID"=w861) -> ("error out"=w854:errorcluster, "Fixed Output Voltage out"=w855:dbl)  [unwired: 4 in, 2 out]
                        n375 = local write "Fixed DC 3"(w855) -> ()
                      }
                      event "Reset Error 3": Value Change {
                        n376 = event-data() -> ()  [unwired: 1 in, 1 out]
                        n377 = local write "Error Message 3"("" ("Error Message 3")) -> ()
                        n378 = local write "Error 3"(FALSE ("Error 3")) -> ()
                      }
                      event "Positioner 3": Value Change {
                        n379 = event-data() -> ()  [unwired: 1 in, 1 out]
                        n380 = property on="Positioner 3" class="MDér (strict)"() -> ("RingText.Text"=w868:string)  [unwired: 2 in, 2 out]
                        n381 = call "controlActorSelection.vi"("Positioner in"=w868, "axis in"=w869, "connection ID"=w870) -> ("error out"=w871:errorcluster, "axis out"=w872:u8, "connection ID"=w873:refnum<k5>)  [unwired: 6 in]
                        n382 = call "getActorType.vi"("error in"=w871, "axis in"=w872, "connection ID"=w873) -> ("error out"=w867:errorcluster, "Actor Type"=w866:dbl)  [unwired: 5 in, 2 out]
                        n383 = local write "actor type 3"(w866) -> ()
                      }
                      event "Target Range 3": Value Change {
                        n384 = event-data() -> ()  [unwired: 1 in, 1 out]
                        n385 = call "controlTargetRange.vi"("Set"=TRUE, "Target Range in"="Target Range 3", "axis in"=w877, "connection ID"=w878) -> ("error out"=w880:errorcluster, "axis out"=w881:u8, "connection ID"=w882:refnum<k5>)  [unwired: 4 in, 1 out]
                        n386 = call "controlTargetRange.vi"("Set"=FALSE, "error in"=w880, "axis in"=w881, "connection ID"=w882) -> ("error out"=w874:errorcluster, "Target Range out"=w875:dbl)  [unwired: 4 in, 2 out]
                        n387 = local write "Target Range 3"(w875) -> ()
                      }
                      event "auto Reset 3": Value Change {
                        n388 = event-data() -> ()  [unwired: 1 in, 1 out]
                        n389 = call "controlAutoReset.vi"("Set"=TRUE, "auto reset in"="auto Reset 3", "axis in"=w888, "connection ID"=w889) -> ("error out"=w885:errorcluster, "axis out"=w891:u8, "connection ID"=w892:refnum<k5>)  [unwired: 4 in, 1 out]
                        n390 = call "controlAutoReset.vi"("Set"=FALSE, "error in"=w885, "axis in"=w891, "connection ID"=w892) -> ("error out"=w884:errorcluster, "auto reset out"=w886:bool)  [unwired: 4 in, 2 out]
                        n391 = local write "auto Reset 3"(w886) -> ()
                      }
                      event "Reference Auto Update 3": Value Change {
                        n392 = event-data() -> ()  [unwired: 1 in, 1 out]
                        n393 = call "controlReferenceAutoUpdate.vi"("Set"=TRUE, "ref auto up in"="Reference Auto Update 3", "axis in"=w896, "connection ID"=w898) -> ("error out"=w899:errorcluster, "axis out"=w900:u8, "connection ID"=w901:refnum<k5>)  [unwired: 4 in, 1 out]
                        n394 = call "controlReferenceAutoUpdate.vi"("Set"=FALSE, "error in"=w899, "axis in"=w900, "connection ID"=w901) -> ("error out"=w894:errorcluster, "ref auto up out"=w895:bool)  [unwired: 4 in, 2 out]
                        n395 = local write "Reference Auto Update 3"(w895) -> ()
                      }
                      event Timeout {
                        n396 = event-data() -> ()  [unwired: 1 in, 1 out]
                        n397 = call "getPosition.vi"("axis in"=w924, "connection ID"=w925) -> ("error out"=w923:errorcluster, "position out"=→"Position 3":dbl, "axis out"=w939:u8, "connection ID"=w940:refnum<k5>)  [unwired: 6 in]
                        n398 = call "getReferencePosition.vi"("error in"=w923, "axis in"=w939, "connection ID"=w940) -> ("error out"=w922:errorcluster, "Reference position out"=→"Reference 3":dbl, "axis out"=w937:u8, "connection ID"=w938:refnum<k5>)  [unwired: 5 in]
                        n399 = call "getStatusConnected.vi"("error in"=w922, "axis in"=w937, "connection ID"=w938) -> ("error out"=w921:errorcluster, "Status Connected out"=→"Connected 3":bool, "axis out"=w935:u8, "connection ID"=w936:refnum<k5>)  [unwired: 5 in]
                        n400 = call "getStatusMoving.vi"("error in"=w921, "axis in"=w935, "connection ID"=w936) -> ("error out"=w920:errorcluster, "status moving out"=→"MoveSignal 3":bool, "axis out"=w933:u8, "connection ID"=w934:refnum<k5>)  [unwired: 5 in]
                        n401 = call "getStatusReference.vi"("error in"=w920, "axis in"=w933, "connection ID"=w934) -> ("error out"=w919:errorcluster, "status reference out"=→"ReferenceSignal 3":bool, "axis out"=w931:u8, "connection ID"=w932:refnum<k5>)  [unwired: 5 in]
                        n402 = call "getStatusEotBkwd.vi"("error in"=w919, "axis in"=w931, "connection ID"=w932) -> ("error out"=w918:errorcluster, "Get Stus EOT BKWD out"=→"EotLeftDetected3":bool, "axis out"=w929:u8, "connection ID"=w930:refnum<k5>)  [unwired: 5 in]
                        n403 = call "getStatusEotFwd.vi"("error in"=w918, "axis in"=w929, "connection ID"=w930) -> ("error out"=w926:errorcluster, "Status EOT FWD out"=→"EotrightDetected3":bool, "axis out"=w927:u8, "connection ID"=w928:refnum<k5>)  [unwired: 5 in]
                        n404 = call "getStatusTargetRange.vi"("error in"=w926, "axis in"=w927, "connection ID"=w928) -> ("error out"=w907:errorcluster, "Status Target Range out"=→"in target range3":bool, "axis out"=w908:u8, "connection ID"=w909:refnum<k5>)  [unwired: 5 in]
                        n405 = call "controlMove.vi"("Set"=FALSE, "error in"=w907, "axis in"=w908, "connection ID"=w909) -> ("error out"=w906:errorcluster, "controll move out"=w904:bool)  [unwired: 4 in, 2 out]
                        n406 = local write "move out 3"(w904) -> ()
                        n407 = local write "Move 3"(w904) -> ()
                      }
                    }
                    n408 = Unbundle(w754) -> ("code"=w753:i32, "source"=w755:string)  [unwired: 1 out]
                    n409 = Not Equal To 0?(x=w753) -> (x != 0?=w752:bool)
                    n410 = case shown="Faux" w752 {
                      selector: w752 -> [_ w758]
                      tunnel: w755 -> [_ w759]
                      frame False {
                      }
                      frame True {
                        "Error Message 3" <- w759
                        "Error 3" <- w758
                      }
                    }
                  }
                }
              }
              frame "Interface" {
                n411 = stacked-sequence {
                  tunnel: w941 -> [w942 w1067 w1192]
                  frame #0 {
                    w948 = u8 0 items=["1", "2", "3"] ("axis in")
                    n412 = event shown="[0] Timeout" {
                      selector: _ -> [_ _ _ _ _ _ _ _ _ _ _]
                      dyn-events: _ -> [_ _ _ _ _ _ _ _ _ _ _]
                      timeout: 10 -> [_ _ _ _ _ _ _ _ _ _ _]
                      tunnel: w948 -> [w958 w982 w993 w1002 w1012 w1020 w1029 w1042 w1050 w1060 _]
                      tunnel: [_ w977 w988 w996 w1009 w1016 w1025 w1037 w1045 w1057 _] -> w945
                      tunnel: w942 -> [w959 w984 w994 w1004 w1014 w1024 w1034 w1044 w1054 w1064 _]
                      event Timeout {
                        n413 = event-data() -> ()  [unwired: 1 in, 1 out]
                        n414 = call "controlRealtimeInputMode.vi"("Set"=FALSE ("set"), "axis in"=w958, "connection ID"=w959) -> ("error out"=w951:errorcluster, "RT Mode out"=w956:i32, "axis out"=w952:u8, "connection ID"=w953:refnum<k5>)  [unwired: 5 in]
                        n415 = local write "Mode Input 1"(w956) -> ()
                        n416 = Equal?(x=w956, y=15) -> (x = y?=w962:bool)
                        n417 = call "controlRealtimeInputLoopMode.vi"("Set"=FALSE ("set"), "error in"=w951, "axis in"=w952, "connection ID"=w953) -> ("RT Loop out"=w955:i32)  [unwired: 4 in, 3 out]
                        n418 = local write "Loop Mode 1"(w955) -> ()
                        n419 = Equal?(x=w955, y=0) -> (x = y?=w960:bool)
                        n420 = case shown="Vrai" w962 {
                          tunnel: w960 -> [w964 _]
                          frame False {
                            n421 = case shown="Vrai" w964 {
                              frame False {
                                w965 = T1."Enabled" ("Disabled")
                                n422 = property on="RT in move 1" class="Bool (strict)"("DisabledEnum"=w965) -> ()  [unwired: 2 in, 2 out]
                                n423 = property on="RT in move Signal 1" class="Bool (strict)"("DisabledEnum"=w965) -> ()  [unwired: 2 in, 2 out]
                                n424 = property on="Loop Mode 1" class="MDér (strict)"("DisabledEnum"=w965) -> ()  [unwired: 2 in, 2 out]
                                n425 = property on="Steps per pulse 1" class="NumNb (strict)"("DisabledEnum"=T1."Disabled and Grayed Out" ("Disabled")) -> ()  [unwired: 2 in, 2 out]
                                n426 = property on="Change per pulse 1" class="NumNb (strict)"("DisabledEnum"=w965) -> ()  [unwired: 2 in, 2 out]
                              }
                              frame True {
                                w968 = T1."Enabled" ("Disabled")
                                w967 = T1."Disabled and Grayed Out" ("Disabled")
                                n427 = property on="RT in move 1" class="Bool (strict)"("DisabledEnum"=w967) -> ()  [unwired: 2 in, 2 out]
                                n428 = property on="RT in move Signal 1" class="Bool (strict)"("DisabledEnum"=w967) -> ()  [unwired: 2 in, 2 out]
                                n429 = property on="Loop Mode 1" class="MDér (strict)"("DisabledEnum"=w968) -> ()  [unwired: 2 in, 2 out]
                                n430 = property on="Steps per pulse 1" class="NumNb (strict)"("DisabledEnum"=w968) -> ()  [unwired: 2 in, 2 out]
                                n431 = property on="Change per pulse 1" class="NumNb (strict)"("DisabledEnum"=w967) -> ()  [unwired: 2 in, 2 out]
                              }
                            }
                          }
                          frame True {
                            w969 = T1."Disabled and Grayed Out" ("Disabled")
                            n432 = property on="RT in move 1" class="Bool (strict)"("DisabledEnum"=w969) -> ()  [unwired: 2 in, 2 out]
                            n433 = property on="RT in move Signal 1" class="Bool (strict)"("DisabledEnum"=w969) -> ()  [unwired: 2 in, 2 out]
                            n434 = property on="Loop Mode 1" class="MDér (strict)"("DisabledEnum"=w969) -> ()  [unwired: 2 in, 2 out]
                            n435 = property on="Steps per pulse 1" class="NumNb (strict)"("DisabledEnum"=w969) -> ()  [unwired: 2 in, 2 out]
                            n436 = property on="Change per pulse 1" class="NumNb (strict)"("DisabledEnum"=w969) -> ()  [unwired: 2 in, 2 out]
                          }
                        }
                      }
                      event "Mode Input 1": Value Change {
                        n437 = event-data() -> ()  [unwired: 1 in, 1 out]
                        n438 = call "controlRealtimeInputMode.vi"("Set"=TRUE, "RT Mode in"="Mode Input 1", "axis in"=w982, "connection ID"=w984) -> ("error out"=w978:errorcluster, "axis out"=w981:u8, "connection ID"=w983:refnum<k5>)  [unwired: 4 in, 1 out]
                        n439 = call "controlRealtimeInputMode.vi"("Set"=FALSE, "error in"=w978, "axis in"=w981, "connection ID"=w983) -> ("error out"=w971:errorcluster, "RT Mode out"=w973:i32, "axis out"=w975:u8, "connection ID"=w976:refnum<k5>)  [unwired: 4 in]
                        n440 = local write "Mode Input 1"(w973) -> ()
                        n441 = call "controlRealtimeInputLoopMode.vi"("Set"=FALSE, "error in"=w971, "axis in"=w975, "connection ID"=w976) -> ("error out"=w977:errorcluster, "RT Loop out"=w972:i32)  [unwired: 4 in, 2 out]
                        n442 = local write "Loop Mode 1"(w972) -> ()
                      }
                      event "Loop Mode 1": Value Change {
                        n443 = event-data() -> ()  [unwired: 1 in, 1 out]
                        n444 = call "controlRealtimeInputLoopMode.vi"("Set"=TRUE, "RT Loop in"="Loop Mode 1", "axis in"=w993, "connection ID"=w994) -> ("error out"=w989:errorcluster, "axis out"=w990:u8, "connection ID"=w991:refnum<k5>)  [unwired: 4 in, 1 out]
                        n445 = call "controlRealtimeInputLoopMode.vi"("Set"=FALSE, "error in"=w989, "axis in"=w990, "connection ID"=w991) -> ("error out"=w988:errorcluster, "RT Loop out"=w986:i32)  [unwired: 4 in, 2 out]
                        n446 = local write "Loop Mode 1"(w986) -> ()
                      }
                      event "Steps per pulse 1": Value Change {
                        n447 = event-data() -> ()  [unwired: 1 in, 1 out]
                        n448 = call "controlRealtimeInputStepsPerPulse.vi"("Set"=TRUE, "Steps in"="Steps per pulse 1", "axis in"=w1002, "connection ID"=w1004) -> ("error out"=w997:errorcluster, "axis out"=w998:u8, "connection ID"=w1003:refnum<k5>)  [unwired: 4 in, 1 out]
                        n449 = call "controlRealtimeInputStepsPerPulse.vi"("Set"=FALSE, "error in"=w997, "axis in"=w998, "connection ID"=w1003) -> ("error out"=w996:errorcluster, "Steps out"=w995:i32)  [unwired: 4 in, 2 out]
                        n450 = local write "Steps per pulse 1"(w995) -> ()
                      }
                      event "Change per pulse 1": Value Change {
                        n451 = event-data() -> ()  [unwired: 1 in, 1 out]
                        n452 = call "controlRealTimeInChangePerPulse.vi"("Set"=TRUE, "Change in"="Change per pulse 1", "axis in"=w1012, "connection ID"=w1014) -> ("error out"=w1010:errorcluster, "axis out"=w1008:u8, "connection ID"=w1013:refnum<k5>)  [unwired: 4 in, 1 out]
                        n453 = call "controlRealTimeInChangePerPulse.vi"("Set"=FALSE, "error in"=w1010, "axis in"=w1008, "connection ID"=w1013) -> ("error out"=w1009:errorcluster, "Change out"=w1007:i32)  [unwired: 4 in, 2 out]
                        n454 = local write "Change per pulse 1"(w1007) -> ()
                      }
                      event "RT in move 1": Value Change {
                        n455 = event-data() -> ()  [unwired: 1 in, 1 out]
                        n456 = call "controlRealtimeInputMove.vi"("Set"=TRUE, "move in"="RT in move 1", "axis in"=w1020, "connection ID"=w1024) -> ("error out"=w1017:errorcluster, "axis out"=w1018:u8, "connection ID"=w1023:refnum<k5>)  [unwired: 4 in, 1 out]
                        n457 = call "controlRealtimeInputMove.vi"("Set"=FALSE, "error in"=w1017, "axis in"=w1018, "connection ID"=w1023) -> ("error out"=w1016:errorcluster, "move out"=→"RT in move Signal 1":bool)  [unwired: 4 in, 2 out]
                      }
                      event "AquadB in res 1": Value Change {
                        n458 = event-data() -> ()  [unwired: 1 in, 1 out]
                        n459 = call "controlAQuadBInResolution.vi"("Set"=TRUE, "Resolution in"="AquadB in res 1", "axis in"=w1029, "connection ID"=w1034) -> ("error out"=w1026:errorcluster, "axis out"=w1032:u8, "connection ID"=w1033:refnum<k5>)  [unwired: 3 in, 1 out]
                        n460 = call "controlAQuadBInResolution.vi"("Set"=FALSE, "error in"=w1026, "axis in"=w1032, "connection ID"=w1033) -> ("error out"=w1025:errorcluster, "Resolution out"=w1027:i32)  [unwired: 3 in, 2 out]
                        n461 = local write "AquadB in res 1"(w1027) -> ()
                      }
                      event "AquadB out 1": Value Change {
                        n462 = event-data() -> ()  [unwired: 1 in, 1 out]
                        n463 = call "controlAQuadBOut.vi"("Set"=TRUE, "ABout in"="AquadB out 1", "axis in"=w1042, "connection ID"=w1044) -> ("error out"=w1038:errorcluster, "axis out"=w1035:u8, "connection ID"=w1043:refnum<k5>)  [unwired: 4 in, 1 out]
                        n464 = call "controlAQuadBOut.vi"("Set"=FALSE, "error in"=w1038, "axis in"=w1035, "connection ID"=w1043) -> ("error out"=w1037:errorcluster, "ABout out"=w1036:bool)  [unwired: 4 in, 2 out]
                        n465 = local write "AquadB out 1"(w1036) -> ()
                      }
                      event "AqaudB clock 1": Value Change {
                        n466 = event-data() -> ()  [unwired: 1 in, 1 out]
                        n467 = call "controlAQuadBOutClock.vi"("Set"=TRUE, "clock in"="AqaudB clock 1", "axis in"=w1050, "connection ID"=w1054) -> ("error out"=w1047:errorcluster, "axis out"=w1049:u8, "connection ID"=w1053:refnum<k5>)  [unwired: 4 in, 1 out]
                        n468 = call "controlAQuadBOutClock.vi"("Set"=FALSE, "error in"=w1047, "axis in"=w1049, "connection ID"=w1053) -> ("error out"=w1045:errorcluster, "clock out"=w1046:i32)  [unwired: 4 in, 2 out]
                        n469 = local write "AqaudB clock 1"(w1046) -> ()
                      }
                      event "AquadB Resolution 1": Value Change {
                        n470 = event-data() -> ()  [unwired: 1 in, 1 out]
                        n471 = call "controlAQuadBOutResolution.vi"("Set"=TRUE, "ABoutRes in"="AquadB Resolution 1", "axis in"=w1060, "connection ID"=w1064) -> ("error out"=w1058:errorcluster, "axis out"=w1059:u8, "connection ID"=w1063:refnum<k5>)  [unwired: 4 in, 1 out]
                        n472 = call "controlAQuadBOutResolution.vi"("Set"=FALSE, "error in"=w1058, "axis in"=w1059, "connection ID"=w1063) -> ("error out"=w1057:errorcluster, "ABoutRes out"=w1055:i32)  [unwired: 4 in, 2 out]
                        n473 = local write "AquadB Resolution 1"(w1055) -> ()
                      }
                      event "Reset Error 4": Value Change {
                        n474 = event-data() -> ()  [unwired: 1 in, 1 out]
                        n475 = local write "Error Message 4"("" ("Error Message")) -> ()
                        n476 = local write "Error 4"(FALSE ("Error 4")) -> ()
                      }
                    }
                    n477 = Unbundle(w945) -> ("code"=w943:i32, "source"=w944:string)  [unwired: 1 out]
                    n478 = Not Equal To 0?(x=w943) -> (x != 0?=w946:bool)
                    n479 = case shown="Vrai" w946 {
                      selector: w946 -> [_ w949]
                      tunnel: w944 -> [_ w950]
                      frame False {
                      }
                      frame True {
                        "Error Message 4" <- w950
                        "Error 4" <- w949
                      }
                    }
                  }
                  frame #1 {
                    w1073 = u8 1 items=["1", "2", "3"] ("axis in")
                    n480 = event shown="[4] \"Change per pulse 2\": Valeur changée" {
                      selector: _ -> [_ _ _ _ _ _ _ _ _ _ _]
                      dyn-events: _ -> [_ _ _ _ _ _ _ _ _ _ _]
                      timeout: 1 -> [_ _ _ _ _ _ _ _ _ _ _]
                      tunnel: w1073 -> [w1082 w1101 w1112 w1123 w1135 w1142 w1152 w1163 w1172 w1182 _]
                      tunnel: [_ w1095 w1114 w1121 w1130 w1143 w1153 w1164 w1173 w1183 _] -> w1068
                      tunnel: w1067 -> [w1083 w1102 w1115 w1124 w1136 w1144 w1154 w1165 w1174 w1184 _]
                      event Timeout {
                        n481 = event-data() -> ()  [unwired: 1 in, 1 out]
                        n482 = call "controlRealtimeInputMode.vi"("Set"=FALSE ("set"), "axis in"=w1082, "connection ID"=w1083) -> ("error out"=w1076:errorcluster, "RT Mode out"=w1081:i32, "axis out"=w1077:u8, "connection ID"=w1078:refnum<k5>)  [unwired: 5 in]
                        n483 = local write "Mode Input 2"(w1081) -> ()
                        n484 = Equal?(x=w1081, y=15) -> (x = y?=w1087:bool)
                        n485 = call "controlRealtimeInputLoopMode.vi"("Set"=FALSE ("set"), "error in"=w1076, "axis in"=w1077, "connection ID"=w1078) -> ("RT Loop out"=w1080:i32)  [unwired: 4 in, 3 out]
                        n486 = local write "Loop Mode 2"(w1080) -> ()
                        n487 = Equal?(x=w1080, y=0) -> (x = y?=w1085:bool)
                        n488 = case shown="Faux" w1087 {
                          tunnel: w1085 -> [w1089 _]
                          frame False {
                            n489 = case shown="Faux" w1089 {
                              frame False {
                                w1090 = T1."Enabled" ("Disabled")
                                n490 = property on="RT in move 2" class="Bool (strict)"("DisabledEnum"=w1090) -> ()  [unwired: 2 in, 2 out]
                                n491 = property on="RT in move Signal 2" class="Bool (strict)"("DisabledEnum"=w1090) -> ()  [unwired: 2 in, 2 out]
                                n492 = property on="Loop Mode 2" class="MDér (strict)"("DisabledEnum"=w1090) -> ()  [unwired: 2 in, 2 out]
                                n493 = property on="Steps per pulse 2" class="NumNb (strict)"("DisabledEnum"=T1."Disabled and Grayed Out" ("Disabled")) -> ()  [unwired: 2 in, 2 out]
                                n494 = property on="Change per pulse 2" class="NumNb (strict)"("DisabledEnum"=w1090) -> ()  [unwired: 2 in, 2 out]
                              }
                              frame True {
                                w1093 = T1."Enabled" ("Disabled")
                                w1092 = T1."Disabled and Grayed Out" ("Disabled")
                                n495 = property on="RT in move 2" class="Bool (strict)"("DisabledEnum"=w1092) -> ()  [unwired: 2 in, 2 out]
                                n496 = property on="RT in move Signal 2" class="Bool (strict)"("DisabledEnum"=w1092) -> ()  [unwired: 2 in, 2 out]
                                n497 = property on="Loop Mode 2" class="MDér (strict)"("DisabledEnum"=w1093) -> ()  [unwired: 2 in, 2 out]
                                n498 = property on="Steps per pulse 2" class="NumNb (strict)"("DisabledEnum"=w1093) -> ()  [unwired: 2 in, 2 out]
                                n499 = property on="Change per pulse 2" class="NumNb (strict)"("DisabledEnum"=w1092) -> ()  [unwired: 2 in, 2 out]
                              }
                            }
                          }
                          frame True {
                            w1094 = T1."Disabled and Grayed Out" ("Disabled")
                            n500 = property on="RT in move 2" class="Bool (strict)"("DisabledEnum"=w1094) -> ()  [unwired: 2 in, 2 out]
                            n501 = property on="RT in move Signal 2" class="Bool (strict)"("DisabledEnum"=w1094) -> ()  [unwired: 2 in, 2 out]
                            n502 = property on="Loop Mode 2" class="MDér (strict)"("DisabledEnum"=w1094) -> ()  [unwired: 2 in, 2 out]
                            n503 = property on="Steps per pulse 2" class="NumNb (strict)"("DisabledEnum"=w1094) -> ()  [unwired: 2 in, 2 out]
                            n504 = property on="Change per pulse 2" class="NumNb (strict)"("DisabledEnum"=w1094) -> ()  [unwired: 2 in, 2 out]
                          }
                        }
                      }
                      event "Mode Input 2": Value Change {
                        n505 = event-data() -> ()  [unwired: 1 in, 1 out]
                        n506 = call "controlRealtimeInputMode.vi"("Set"=TRUE, "RT Mode in"="Mode Input 2", "axis in"=w1101, "connection ID"=w1102) -> ("error out"=w1097:errorcluster, "axis out"=w1107:u8, "connection ID"=w1109:refnum<k5>)  [unwired: 4 in, 1 out]
                        n507 = call "controlRealtimeInputMode.vi"("Set"=FALSE, "error in"=w1097, "axis in"=w1107, "connection ID"=w1109) -> ("error out"=w1096:errorcluster, "RT Mode out"=w1099:i32, "axis out"=w1106:u8, "connection ID"=w1108:refnum<k5>)  [unwired: 4 in]
                        n508 = local write "Mode Input 2"(w1099) -> ()
                        n509 = call "controlRealtimeInputLoopMode.vi"("Set"=FALSE, "error in"=w1096, "axis in"=w1106, "connection ID"=w1108) -> ("error out"=w1095:errorcluster, "RT Loop out"=w1098:i32)  [unwired: 4 in, 2 out]
                        n510 = local write "Loop Mode 2"(w1098) -> ()
                      }
                      event "Loop Mode 2": Value Change {
                        n511 = event-data() -> ()  [unwired: 1 in, 1 out]
                        n512 = call "controlRealtimeInputLoopMode.vi"("Set"=TRUE, "RT Loop in"="Loop Mode 2", "axis in"=w1112, "connection ID"=w1115) -> ("error out"=w1116:errorcluster, "axis out"=w1117:u8, "connection ID"=w1118:refnum<k5>)  [unwired: 4 in, 1 out]
                        n513 = call "controlRealtimeInputLoopMode.vi"("Set"=FALSE, "error in"=w1116, "axis in"=w1117, "connection ID"=w1118) -> ("error out"=w1114:errorcluster, "RT Loop out"=w1111:i32)  [unwired: 4 in, 2 out]
                        n514 = local write "Loop Mode 2"(w1111) -> ()
                      }
                      event "Steps per pulse 2": Value Change {
                        n515 = event-data() -> ()  [unwired: 1 in, 1 out]
                        n516 = call "controlRealtimeInputStepsPerPulse.vi"("Set"=TRUE, "Steps in"="Steps per pulse 2", "axis in"=w1123, "connection ID"=w1124) -> ("error out"=w1125:errorcluster, "axis out"=w1126:u8, "connection ID"=w1129:refnum<k5>)  [unwired: 4 in, 1 out]
                        n517 = call "controlRealtimeInputStepsPerPulse.vi"("Set"=FALSE, "error in"=w1125, "axis in"=w1126, "connection ID"=w1129) -> ("error out"=w1121:errorcluster, "Steps out"=w1120:i32)  [unwired: 4 in, 2 out]
                        n518 = local write "Steps per pulse 2"(w1120) -> ()
                      }
                      event "Change per pulse 2": Value Change {
                        n519 = event-data() -> ()  [unwired: 1 in, 1 out]
                        n520 = call "controlRealTimeInChangePerPulse.vi"("Set"=TRUE, "Change in"="Change per pulse 2", "axis in"=w1135, "connection ID"=w1136) -> ("error out"=w1138:errorcluster, "axis out"=w1137:u8, "connection ID"=w1139:refnum<k5>)  [unwired: 4 in, 1 out]
                        n521 = call "controlRealTimeInChangePerPulse.vi"("Set"=FALSE, "error in"=w1138, "axis in"=w1137, "connection ID"=w1139) -> ("error out"=w1130:errorcluster, "Change out"=w1131:i32)  [unwired: 4 in, 2 out]
                        n522 = local write "Change per pulse 2"(w1131) -> ()
                      }
                      event "RT in move 2": Value Change {
                        n523 = event-data() -> ()  [unwired: 1 in, 1 out]
                        n524 = call "controlRealtimeInputMove.vi"("Set"=TRUE, "move in"="RT in move 2", "axis in"=w1142, "connection ID"=w1144) -> ("error out"=w1145:errorcluster, "axis out"=w1146:u8, "connection ID"=w1149:refnum<k5>)  [unwired: 4 in, 1 out]
                        n525 = call "controlRealtimeInputMove.vi"("Set"=FALSE, "error in"=w1145, "axis in"=w1146, "connection ID"=w1149) -> ("error out"=w1143:errorcluster, "move out"=→"RT in move Signal 2":bool)  [unwired: 4 in, 2 out]
                      }
                      event "AquadB in res 2": Value Change {
                        n526 = event-data() -> ()  [unwired: 1 in, 1 out]
                        n527 = call "controlAQuadBInResolution.vi"("Set"=TRUE, "Resolution in"="AquadB in res 2", "axis in"=w1152, "connection ID"=w1154) -> ("error out"=w1155:errorcluster, "axis out"=w1158:u8, "connection ID"=w1159:refnum<k5>)  [unwired: 3 in, 1 out]
                        n528 = call "controlAQuadBInResolution.vi"("Set"=FALSE, "error in"=w1155, "axis in"=w1158, "connection ID"=w1159) -> ("error out"=w1153:errorcluster, "Resolution out"=w1150:i32)  [unwired: 3 in, 2 out]
                        n529 = local write "AquadB in res 2"(w1150) -> ()
                      }
                      event "AquadB out 2": Value Change {
                        n530 = event-data() -> ()  [unwired: 1 in, 1 out]
                        n531 = call "controlAQuadBOut.vi"("Set"=TRUE, "ABout in"="AquadB out 2", "axis in"=w1163, "connection ID"=w1165) -> ("error out"=w1166:errorcluster, "axis out"=w1162:u8, "connection ID"=w1169:refnum<k5>)  [unwired: 4 in, 1 out]
                        n532 = call "controlAQuadBOut.vi"("Set"=FALSE, "error in"=w1166, "axis in"=w1162, "connection ID"=w1169) -> ("error out"=w1164:errorcluster, "ABout out"=w1160:bool)  [unwired: 4 in, 2 out]
                        n533 = local write "AquadB out 2"(w1160) -> ()
                      }
                      event "AqaudB clock 2": Value Change {
                        n534 = event-data() -> ()  [unwired: 1 in, 1 out]
                        n535 = call "controlAQuadBOutClock.vi"("Set"=TRUE, "clock in"="AqaudB clock 2", "axis in"=w1172, "connection ID"=w1174) -> ("error out"=w1175:errorcluster, "axis out"=w1176:u8, "connection ID"=w1179:refnum<k5>)  [unwired: 4 in, 1 out]
                        n536 = call "controlAQuadBOutClock.vi"("Set"=FALSE, "error in"=w1175, "axis in"=w1176, "connection ID"=w1179) -> ("error out"=w1173:errorcluster, "clock out"=w1170:i32)  [unwired: 4 in, 2 out]
                        n537 = local write "AqaudB clock 2"(w1170) -> ()
                      }
                      event "AquadB Resolution 2": Value Change {
                        n538 = event-data() -> ()  [unwired: 1 in, 1 out]
                        n539 = call "controlAQuadBOutResolution.vi"("Set"=TRUE, "ABoutRes in"="AquadB Resolution 2", "axis in"=w1182, "connection ID"=w1184) -> ("error out"=w1185:errorcluster, "axis out"=w1186:u8, "connection ID"=w1189:refnum<k5>)  [unwired: 4 in, 1 out]
                        n540 = call "controlAQuadBOutResolution.vi"("Set"=FALSE, "error in"=w1185, "axis in"=w1186, "connection ID"=w1189) -> ("error out"=w1183:errorcluster, "ABoutRes out"=w1180:i32)  [unwired: 4 in, 2 out]
                        n541 = local write "AquadB Resolution 2"(w1180) -> ()
                      }
                      event "Reset Error 5": Value Change {
                        n542 = event-data() -> ()  [unwired: 1 in, 1 out]
                        n543 = local write "Error 5"(FALSE ("Error 5")) -> ()
                        n544 = local write "Error Message 5"("" ("Error Message")) -> ()
                      }
                    }
                    n545 = Unbundle(w1068) -> ("code"=w1070:i32, "source"=w1069:string)  [unwired: 1 out]
                    n546 = Not Equal To 0?(x=w1070) -> (x != 0?=w1071:bool)
                    n547 = case shown="Vrai" w1071 {
                      selector: w1071 -> [_ w1074]
                      tunnel: w1069 -> [_ w1075]
                      frame False {
                      }
                      frame True {
                        "Error Message 5" <- w1075
                        "Error 5" <- w1074
                      }
                    }
                  }
                  frame #2 {
                    w1197 = u8 2 items=["1", "2", "3"] ("axis in")
                    n548 = event shown="[8] \"AquadB out 3\": Valeur changée" {
                      selector: _ -> [_ _ _ _ _ _ _ _ _ _ _ _]
                      dyn-events: _ -> [_ _ _ _ _ _ _ _ _ _ _ _]
                      timeout: 1 -> [_ _ _ _ _ _ _ _ _ _ _ _]
                      tunnel: w1197 -> [w1207 w1222 w1239 w1248 w1257 w1267 w1278 _ w1296 w1306 w1316 _]
                      tunnel: [_ w1224 w1236 w1245 w1258 w1268 w1277 w1286 w1293 w1303 w1313 _] -> w1193
                      tunnel: w1192 -> [w1208 w1227 w1240 w1249 w1259 w1269 w1279 w1292 w1297 w1307 w1317 _]
                      event Timeout {
                        n549 = event-data() -> ()  [unwired: 1 in, 1 out]
                        n550 = call "controlRealtimeInputMode.vi"("Set"=FALSE ("set"), "axis in"=w1207, "connection ID"=w1208) -> ("error out"=w1201:errorcluster, "RT Mode out"=w1206:i32, "axis out"=w1202:u8, "connection ID"=w1203:refnum<k5>)  [unwired: 5 in]
                        n551 = local write "Mode Input 3"(w1206) -> ()
                        n552 = Equal?(x=w1206, y=15) -> (x = y?=w1212:bool)
                        n553 = call "controlRealtimeInputLoopMode.vi"("Set"=FALSE ("set"), "error in"=w1201, "axis in"=w1202, "connection ID"=w1203) -> ("RT Loop out"=w1205:i32)  [unwired: 4 in, 3 out]
                        n554 = local write "Loop Mode 3"(w1205) -> ()
                        n555 = Equal?(x=w1205, y=0) -> (x = y?=w1210:bool)
                        n556 = case shown="Faux" w1212 {
                          tunnel: w1210 -> [w1214 _]
                          frame False {
                            n557 = case shown="Vrai" w1214 {
                              frame False {
                                w1215 = T1."Enabled" ("Disabled")
                                n558 = property on="RT in move 3" class="Bool (strict)"("DisabledEnum"=w1215) -> ()  [unwired: 2 in, 2 out]
                                n559 = property on="RT in move Signal 3" class="Bool (strict)"("DisabledEnum"=w1215) -> ()  [unwired: 2 in, 2 out]
                                n560 = property on="Loop Mode 3" class="MDér (strict)"("DisabledEnum"=w1215) -> ()  [unwired: 2 in, 2 out]
                                n561 = property on="Steps per pulse 3" class="NumNb (strict)"("DisabledEnum"=T1."Disabled and Grayed Out" ("Disabled")) -> ()  [unwired: 2 in, 2 out]
                                n562 = property on="Change per pulse 3" class="NumNb (strict)"("DisabledEnum"=w1215) -> ()  [unwired: 2 in, 2 out]
                              }
                              frame True {
                                w1218 = T1."Enabled" ("Disabled")
                                w1217 = T1."Disabled and Grayed Out" ("Disabled")
                                n563 = property on="RT in move 3" class="Bool (strict)"("DisabledEnum"=w1217) -> ()  [unwired: 2 in, 2 out]
                                n564 = property on="RT in move Signal 3" class="Bool (strict)"("DisabledEnum"=w1217) -> ()  [unwired: 2 in, 2 out]
                                n565 = property on="Loop Mode 3" class="MDér (strict)"("DisabledEnum"=w1218) -> ()  [unwired: 2 in, 2 out]
                                n566 = property on="Steps per pulse 3" class="NumNb (strict)"("DisabledEnum"=w1218) -> ()  [unwired: 2 in, 2 out]
                                n567 = property on="Change per pulse 3" class="NumNb (strict)"("DisabledEnum"=w1217) -> ()  [unwired: 2 in, 2 out]
                              }
                            }
                          }
                          frame True {
                            w1219 = T1."Disabled and Grayed Out" ("Disabled")
                            n568 = property on="RT in move 3" class="Bool (strict)"("DisabledEnum"=w1219) -> ()  [unwired: 2 in, 2 out]
                            n569 = property on="RT in move Signal 3" class="Bool (strict)"("DisabledEnum"=w1219) -> ()  [unwired: 2 in, 2 out]
                            n570 = property on="Loop Mode 3" class="MDér (strict)"("DisabledEnum"=w1219) -> ()  [unwired: 2 in, 2 out]
                            n571 = property on="Steps per pulse 3" class="NumNb (strict)"("DisabledEnum"=w1219) -> ()  [unwired: 2 in, 2 out]
                            n572 = property on="Change per pulse 3" class="NumNb (strict)"("DisabledEnum"=w1219) -> ()  [unwired: 2 in, 2 out]
                          }
                        }
                      }
                      event "Mode Input 3": Value Change {
                        n573 = event-data() -> ()  [unwired: 1 in, 1 out]
                        n574 = call "controlRealtimeInputMode.vi"("Set"=TRUE, "RT Mode in"="Mode Input 3", "axis in"=w1222, "connection ID"=w1227) -> ("error out"=w1226:errorcluster, "axis out"=w1232:u8, "connection ID"=w1234:refnum<k5>)  [unwired: 4 in, 1 out]
                        n575 = call "controlRealtimeInputMode.vi"("Set"=FALSE, "error in"=w1226, "axis in"=w1232, "connection ID"=w1234) -> ("error out"=w1225:errorcluster, "RT Mode out"=w1221:i32, "axis out"=w1231:u8, "connection ID"=w1233:refnum<k5>)  [unwired: 4 in]
                        n576 = local write "Mode Input 3"(w1221) -> ()
                        n577 = call "controlRealtimeInputLoopMode.vi"("Set"=FALSE, "error in"=w1225, "axis in"=w1231, "connection ID"=w1233) -> ("error out"=w1224:errorcluster, "RT Loop out"=w1220:i32)  [unwired: 4 in, 2 out]
                        n578 = local write "Loop Mode 3"(w1220) -> ()
                      }
                      event "Loop Mode 3": Value Change {
                        n579 = event-data() -> ()  [unwired: 1 in, 1 out]
                        n580 = call "controlRealtimeInputLoopMode.vi"("Set"=TRUE, "RT Loop in"="Loop Mode 3", "axis in"=w1239, "connection ID"=w1240) -> ("error out"=w1241:errorcluster, "axis out"=w1242:u8, "connection ID"=w1243:refnum<k5>)  [unwired: 4 in, 1 out]
                        n581 = call "controlRealtimeInputLoopMode.vi"("Set"=FALSE, "error in"=w1241, "axis in"=w1242, "connection ID"=w1243) -> ("error out"=w1236:errorcluster, "RT Loop out"=w1237:i32)  [unwired: 4 in, 2 out]
                        n582 = local write "Loop Mode 3"(w1237) -> ()
                      }
                      event "Steps per pulse 3": Value Change {
                        n583 = event-data() -> ()  [unwired: 1 in, 1 out]
                        n584 = call "controlRealtimeInputStepsPerPulse.vi"("Set"=TRUE, "Steps in"="Steps per pulse 3", "axis in"=w1248, "connection ID"=w1249) -> ("error out"=w1250:errorcluster, "axis out"=w1251:u8, "connection ID"=w1254:refnum<k5>)  [unwired: 4 in, 1 out]
                        n585 = call "controlRealtimeInputStepsPerPulse.vi"("Set"=FALSE, "error in"=w1250, "axis in"=w1251, "connection ID"=w1254) -> ("error out"=w1245:errorcluster, "Steps out"=w1246:i32)  [unwired: 4 in, 2 out]
                        n586 = local write "Steps per pulse 3"(w1246) -> ()
                      }
                      event "Change per pulse 3": Value Change {
                        n587 = event-data() -> ()  [unwired: 1 in, 1 out]
                        n588 = call "controlRealTimeInChangePerPulse.vi"("Set"=TRUE, "Change in"="Change per pulse 3", "axis in"=w1257, "connection ID"=w1259) -> ("error out"=w1263:errorcluster, "axis out"=w1262:u8, "connection ID"=w1264:refnum<k5>)  [unwired: 4 in, 1 out]
                        n589 = call "controlRealTimeInChangePerPulse.vi"("Set"=FALSE, "error in"=w1263, "axis in"=w1262, "connection ID"=w1264) -> ("error out"=w1258:errorcluster, "Change out"=w1255:i32)  [unwired: 4 in, 2 out]
                        n590 = local write "Change per pulse 3"(w1255) -> ()
                      }
                      event "RT in move 3": Value Change {
                        n591 = event-data() -> ()  [unwired: 1 in, 1 out]
                        n592 = call "controlRealtimeInputMove.vi"("Set"=TRUE, "move in"="RT in move 3", "axis in"=w1267, "connection ID"=w1269) -> ("error out"=w1270:errorcluster, "axis out"=w1271:u8, "connection ID"=w1274:refnum<k5>)  [unwired: 4 in, 1 out]
                        n593 = call "controlRealtimeInputMove.vi"("Set"=FALSE, "error in"=w1270, "axis in"=w1271, "connection ID"=w1274) -> ("error out"=w1268:errorcluster, "move out"=→"RT in move Signal 3":bool)  [unwired: 4 in, 2 out]
                      }
                      event "AquadB in res 3": Value Change {
                        n594 = event-data() -> ()  [unwired: 1 in, 1 out]
                        n595 = call "controlAQuadBInResolution.vi"("Set"=TRUE, "Resolution in"="AquadB in res 3", "axis in"=w1278, "connection ID"=w1279) -> ("error out"=w1280:errorcluster, "axis out"=w1283:u8, "connection ID"=w1284:refnum<k5>)  [unwired: 3 in, 1 out]
                        n596 = call "controlAQuadBInResolution.vi"("Set"=FALSE, "error in"=w1280, "axis in"=w1283, "connection ID"=w1284) -> ("error out"=w1277:errorcluster, "Resolution out"=w1275:i32)  [unwired: 3 in, 2 out]
                        n597 = local write "AquadB in res 3"(w1275) -> ()
                      }
                      event "Output Mode": Value Change {
                        n598 = event-data() -> ()  [unwired: 1 in, 1 out]
                        n599 = call "controlRtOutSignalMode.vi"("Set"=TRUE, "RT out Mode in"="Output Mode", "connection ID"=w1292) -> ("error out"=w1287:errorcluster, "connection ID"=w1291:refnum<k5>)  [unwired: 6 in, 1 out]
                        n600 = call "controlRtOutSignalMode.vi"("Set"=FALSE, "error in"=w1287, "connection ID"=w1291) -> ("error out"=w1286:errorcluster, "RT out Mode out"=w1285:i32)  [unwired: 6 in, 1 out]
                        n601 = local write "Output Mode"(w1285) -> ()
                      }
                      event "AquadB out 3": Value Change {
                        n602 = event-data() -> ()  [unwired: 1 in, 1 out]
                        n603 = call "controlAQuadBOut.vi"("Set"=TRUE, "ABout in"="AquadB out 3", "axis in"=w1296, "connection ID"=w1297) -> ("error out"=w1299:errorcluster, "axis out"=w1298:u8, "connection ID"=w1302:refnum<k5>)  [unwired: 4 in, 1 out]
                        n604 = call "controlAQuadBOut.vi"("Set"=FALSE, "error in"=w1299, "axis in"=w1298, "connection ID"=w1302) -> ("error out"=w1293:errorcluster, "ABout out"=w1294:bool)  [unwired: 4 in, 2 out]
                        n605 = local write "AquadB out 3"(w1294) -> ()
                      }
                      event "AqaudB clock 3": Value Change {
                        n606 = event-data() -> ()  [unwired: 1 in, 1 out]
                        n607 = call "controlAQuadBOutClock.vi"("Set"=TRUE, "clock in"="AqaudB clock 3", "axis in"=w1306, "connection ID"=w1307) -> ("error out"=w1308:errorcluster, "axis out"=w1309:u8, "connection ID"=w1312:refnum<k5>)  [unwired: 4 in, 1 out]
                        n608 = call "controlAQuadBOutClock.vi"("Set"=FALSE, "error in"=w1308, "axis in"=w1309, "connection ID"=w1312) -> ("error out"=w1303:errorcluster, "clock out"=w1304:i32)  [unwired: 4 in, 2 out]
                        n609 = local write "AqaudB clock 3"(w1304) -> ()
                      }
                      event "AquadB Resolution 3": Value Change {
                        n610 = event-data() -> ()  [unwired: 1 in, 1 out]
                        n611 = call "controlAQuadBOutResolution.vi"("Set"=TRUE, "ABoutRes in"="AquadB Resolution 3", "axis in"=w1316, "connection ID"=w1317) -> ("error out"=w1318:errorcluster, "axis out"=w1319:u8, "connection ID"=w1322:refnum<k5>)  [unwired: 4 in, 1 out]
                        n612 = call "controlAQuadBOutResolution.vi"("Set"=FALSE, "error in"=w1318, "axis in"=w1319, "connection ID"=w1322) -> ("error out"=w1313:errorcluster, "ABoutRes out"=w1314:i32)  [unwired: 4 in, 2 out]
                        n613 = local write "AquadB Resolution 3"(w1314) -> ()
                      }
                      event "Reset Error 6": Value Change {
                        n614 = event-data() -> ()  [unwired: 1 in, 1 out]
                        n615 = local write "Error 6"(FALSE ("Error 6")) -> ()
                        n616 = local write "Error Message 6"("" ("Error Message")) -> ()
                      }
                    }
                    n617 = Unbundle(w1193) -> ("code"=w1195:i32, "source"=w1196:string)  [unwired: 1 out]
                    n618 = Not Equal To 0?(x=w1195) -> (x != 0?=w1194:bool)
                    n619 = case shown="Vrai" w1194 {
                      selector: w1194 -> [_ w1199]
                      tunnel: w1196 -> [_ w1200]
                      frame False {
                      }
                      frame True {
                        "Error Message 6" <- w1200
                        "Error 6" <- w1199
                      }
                    }
                  }
                }
              }
              frame "About" {
                n620 = event shown="[7] \"Reset Error 8\": Valeur changée" {
                  selector: _ -> [_ _ _ _ _ _ _ _]
                  dyn-events: _ -> [_ _ _ _ _ _ _ _]
                  timeout: 10 -> [_ _ _ _ _ _ _ _]
                  tunnel: w1329 -> [w1339 w1342 w1345 w1347 w1350 w1352 w1354 _]
                  tunnel: [w1335 w1341 w1343 w1346 w1348 w1351 w1353 _] -> w1325
                  event Timeout {
                    n621 = event-data() -> ()  [unwired: 1 in, 1 out]
                    n622 = call "getDeviceName.vi"("connection ID in"=w1339) -> ("error out"=w1336:errorcluster, "Device Name out"=→"Name":string, "connection ID out"=w1337:refnum<k5>)  [unwired: 8 in]
                    n623 = call "getLockStatus.vi"("error in"=w1336, "connection ID in"=w1337) -> ("error out"=w1335:errorcluster, "locked"=→"locked":bool, "authorized"=→"authorized":bool)  [unwired: 6 in, 1 out]
                  }
                  event "name": Value Change {
                    n624 = event-data() -> ()  [unwired: 1 in, 1 out]
                    n625 = call "setDeviceName.vi"("device name in"="name", "connection ID"=w1342) -> ("error out"=w1341:errorcluster)  [unwired: 8 in, 1 out]
                  }
                  event "Lock password": Value Change {
                    n626 = event-data() -> ()  [unwired: 1 in, 1 out]
                    n627 = call "lock.vi"("password"="Lock password", "connection ID"=w1345) -> ("error out"=w1343:errorcluster)  [unwired: 8 in, 1 out]
                  }
                  event "Unlock": Value Change {
                    n628 = event-data() -> ()  [unwired: 1 in, 1 out]
                    n629 = call "unlock.vi"("connection ID"=w1347) -> ("error out"=w1346:errorcluster)  [unwired: 9 in, 1 out]
                  }
                  event "Access Password": Value Change {
                    n630 = event-data() -> ()  [unwired: 1 in, 1 out]
                    n631 = call "grantAccess.vi"("password"="Access Password", "connection ID"=w1350) -> ("error out"=w1348:errorcluster)  [unwired: 8 in, 1 out]
                  }
                  event "Reboot": Value Change {
                    n632 = event-data() -> ()  [unwired: 1 in, 1 out]
                    n633 = call "rebootSystem.vi"("connection ID"=w1352) -> ("error out"=w1351:errorcluster)  [unwired: 9 in, 1 out]
                  }
                  event "Factory Reset": Value Change {
                    n634 = event-data() -> ()  [unwired: 1 in, 1 out]
                    n635 = call "factoryReset.vi"("connection ID"=w1354) -> ("error out"=w1353:errorcluster)  [unwired: 9 in, 1 out]
                  }
                  event "Reset Error 8": Value Change {
                    n636 = event-data() -> ()  [unwired: 1 in, 1 out]
                    n637 = local write "Error 7"(FALSE ("Error 7")) -> ()
                    n638 = local write "Error Message 7"("" ("Error Message 9")) -> ()
                  }
                }
                n639 = Unbundle(w1325) -> ("code"=w1328:i32, "source"=w1326:string)  [unwired: 1 out]
                n640 = Not Equal To 0?(x=w1328) -> (x != 0?=w1327:bool)
                n641 = case shown="Vrai" w1327 {
                  selector: w1327 -> [_ w1332]
                  tunnel: w1326 -> [_ w1331]
                  frame False {
                  }
                  frame True {
                    "Error Message 7" <- w1331
                    "Error 7" <- w1332
                  }
                }
              }
            }
          }
        }
        frame #2 {
          # "Exit / Disconnect"
          n642 = local write "stop"(FALSE ("stop")) -> ()
          n643 = call "close.vi"("connection ID"=w1357) -> ()  [unwired: 6 in, 1 out]
        }
      }
    }
    frame True {
    }
  }
